vi "readLOG.vi"() -> ()   [LabVIEW 2011]
uses:
  <vilib>/Utility/file.llb/Write To Spreadsheet File (DBL).vi
panel:
  in  "save":bool
  out "output cluster":cluster{i32[], dbl[]}[](graph)=[{[0, 1, 2, 3, 4, 5, 6, 7, 8, 9, 10, 11, 12, 13, 14, 15, 16, 17, 18, 19, 20, 21, 22, 23, 24, 25, 26, 27, 28, 29, 30, 31, 32, 33, 34, 35, 36, 37, 38, 39, 40, 41, 42, 43, 44, 45, 46, 47, 48, 49, 50, 51, 52, 53, 54, 55, 56, 57, 58, 59, 60, 61, 62, 63, 64, 65, 66, 67, 68, 69, 70, 71, 72, 73, 74, 75, 76, 77, 78, 79, 80, 81, 82, 83, 84, 85, 86, 87, 88, 89, 90, 91, 92, 93, 94, 95, 96, 97, 98, 99, 100, 101, 102, 103, 104, 105, 106, 107, 108, 109, 110, 111, 112, 113, 114, 115, 116, 117, 118, 119, 120, 121, 122, 123, 124, 125, 126, 127, 128, 129, 130, 131, 132, 133, 134, 135, 136, 137, 138, 139, 140, 141, 142, 143, 144, 145, 146, 147, 148, 149, 150, 151, 152, 153, 154, 155, 156, 157, 158, 159, 160, 161, 162, 163, 164, 165, 166, 167, 168, 169, 170, 171, 172, 173, 174, 175, 176, 177, 178, 179, 180, 181, 182, 183, 184, 185, 186, 187, 188, 189, 190, 191, 192, 193, 194, 195, 196, 197, 198, 199, 200, 201, 202, 203, 204, 205, 206, 207, 208, 209, 210, 211, 212, 213, 214, 215, 216, 217, 218, 219, 220, 221, 222, 223, 224, 225, 226, 227, 228, 229, 230, 231, 232, 233, 234, 235, 236, 237, 238, 239, 240, 241, 242, 243, 244, 245, 246, 247, 248, 249, 250, 251, 252, 253, 254, 255, 256, 257, 258, 259, 260, 261, 262, 263, 264, 265, 266, 267, 268, 269, 270, 271, 272, 273, 274, 275, 276, 277, 278, 279, 280, 281, 282, 283, 284, 285, 286, 287, 288, 289, 290, 291, 292, 293, 294, 295, 296, 297, 298, 299, 300, 301, 302, 303, 304, 305, 306, 307, 308, 309, 310, 311, 312, 313, 314, 315, 316, 317, 318, 319, 320, 321, 322, 323, 324, 325, 326, 327, 328, 329, 330, 331, 332, 333, 334, 335, 336, 337, 338, 339, 340, 341, 342, 343, 344, 345, 346, 347, 348, 349, 350, 351, 352, 353, 354, 355, 356, 357, 358, 359, 360, 361, 362, 363, 364, 365, 366, 367, 368, 369, 370, 371, 372, 373, 374, 375, 376, 377, 378, 379, 380, 381, 382, 383, 384, 385, 386, 387, 388, 389, 390, 391, 392, 393, 394, 395, 396, 397, 398, 399, 400, 401, 402, 403, 404, 405, 406, 407, 408, 409, 410, 411, 412, 413, 414, 415, 416, 417, 418, 419, 420, 421, 422, 423, 424, 425, 426, 427, 428, 429, 430, 431, 432, 433, 434, 435, 436, 437, 438, 439, 440, 441, 442, 443, 444, 445, 446, 447, 448, 449, 450, 451, 452, 453, 454, 455, 456, 457, 458, 459, 460, 461, 462, 463, 464, 465, 466, 467, 468, 469, 470, 471, 472, 473, 474, 475, 476, 477, 478, 479, 480, 481, 482, 483, 484, 485, 486, 487, 488, 489, 490, 491, 492, 493], [nan, nan, nan, nan, nan, nan, nan, nan, nan, nan, nan, nan, nan, nan, nan, nan, nan, nan, nan, nan, nan, nan, nan, nan, nan, nan, nan, nan, nan, nan, nan, nan, nan, nan, nan, nan, nan, nan, nan, nan, nan, nan, nan, nan, nan, nan, nan, nan, nan, nan, nan, nan, nan, nan, nan, nan, nan, nan, nan, nan, nan, nan, nan, nan, nan, nan, nan, nan, nan, nan, nan, nan, nan, nan, nan, nan, nan, nan, nan, nan, nan, nan, nan, nan, nan, nan, nan, nan, nan, nan, nan, nan, nan, nan, nan, nan, nan, nan, nan, nan, nan, nan, nan, nan, nan, nan, nan, nan, nan, nan, nan, nan, nan, nan, nan, nan, nan, nan, nan, nan, nan, nan, nan, nan, nan, nan, nan, nan, nan, nan, nan, nan, nan, nan, nan, nan, nan, nan, nan, nan, nan, nan, nan, nan, nan, nan, nan, nan, nan, nan, nan, nan, nan, nan, nan, nan, nan, nan, nan, nan, nan, nan, nan, nan, nan, nan, nan, nan, nan, nan, nan, nan, nan, nan, nan, nan, nan, nan, nan, nan, nan, nan, nan, nan, nan, nan, nan, nan, nan, nan, nan, nan, nan, nan, nan, nan, nan, nan, nan, nan, nan, nan, nan, nan, nan, nan, nan, nan, nan, nan, nan, nan, nan, nan, nan, nan, nan, nan, nan, nan, nan, nan, nan, nan, nan, nan, nan, nan, nan, nan, nan, nan, nan, nan, nan, nan, nan, nan, nan, nan, nan, nan, nan, nan, nan, nan, nan, nan, nan, nan, nan, nan, nan, nan, nan, nan, nan, nan, nan, nan, nan, nan, nan, nan, nan, nan, nan, nan, nan, nan, nan, nan, nan, nan, nan, nan, nan, nan, nan, nan, nan, nan, nan, nan, nan, nan, nan, nan, nan, nan, nan, nan, nan, nan, nan, nan, nan, nan, nan, nan, nan, nan, nan, nan, nan, nan, nan, nan, nan, nan, nan, nan, nan, nan, nan, nan, nan, nan, nan, nan, nan, nan, nan, nan, nan, nan, nan, nan, nan, nan, nan, nan, nan, nan, nan, nan, nan, nan, nan, nan, nan, nan, nan, nan, nan, nan, nan, nan, nan, nan, nan, nan, nan, nan, nan, nan, nan, nan, nan, nan, nan, nan, nan, nan, nan, nan, nan, nan, nan, nan, nan, nan, nan, nan, nan, nan, nan, nan, nan, nan, nan, nan, nan, nan, nan, nan, nan, nan, nan, nan, nan, nan, nan, nan, nan, nan, nan, nan, nan, nan, nan, nan, nan, nan, nan, nan, nan, nan, nan, nan, nan, nan, nan, nan, nan, nan, nan, nan, nan, nan, nan, nan, nan, nan, nan, nan, nan, nan, nan, nan, nan, nan, nan, nan, nan, nan, nan, nan, nan, nan, nan, nan, nan, nan, nan, nan, nan, nan, nan, nan, nan, nan, nan, nan, nan, nan, nan, nan, nan, nan, nan, nan, nan, nan, nan, nan, nan, nan, nan, nan, nan, nan, nan, nan, nan, nan, nan, nan, nan, nan, nan, nan, nan, nan, nan, nan, nan, nan, nan, nan, nan, nan, nan, nan]}, {[0, 1, 2, 3, 4, 5, 6, 7, 8, 9, 10, 11, 12, 13, 14, 15, 16, 17, 18, 19, 20, 21, 22, 23, 24, 25, 26, 27, 28, 29, 30, 31, 32, 33, 34, 35, 36, 37, 38, 39, 40, 41, 42, 43, 44, 45, 46, 47, 48, 49, 50, 51, 52, 53, 54, 55, 56, 57, 58, 59, 60, 61, 62, 63, 64, 65, 66, 67, 68, 69, 70, 71, 72, 73, 74, 75, 76, 77, 78, 79, 80, 81, 82, 83, 84, 85, 86, 87, 88, 89, 90, 91, 92, 93, 94, 95, 96, 97, 98, 99, 100, 101, 102, 103, 104, 105, 106, 107, 108, 109, 110, 111, 112, 113, 114, 115, 116, 117, 118, 119, 120, 121, 122, 123, 124, 125, 126, 127, 128, 129, 130, 131, 132, 133, 134, 135, 136, 137, 138, 139, 140, 141, 142, 143, 144, 145, 146, 147, 148, 149, 150, 151, 152, 153, 154, 155, 156, 157, 158, 159, 160, 161, 162, 163, 164, 165, 166, 167, 168, 169, 170, 171, 172, 173, 174, 175, 176, 177, 178, 179, 180, 181, 182, 183, 184, 185, 186, 187, 188, 189, 190, 191, 192, 193, 194, 195, 196, 197, 198, 199, 200, 201, 202, 203, 204, 205, 206, 207, 208, 209, 210, 211, 212, 213, 214, 215, 216, 217, 218, 219, 220, 221, 222, 223, 224, 225, 226, 227, 228, 229, 230, 231, 232, 233, 234, 235, 236, 237, 238, 239, 240, 241, 242, 243, 244, 245, 246, 247, 248, 249, 250, 251, 252, 253, 254, 255, 256, 257, 258, 259, 260, 261, 262, 263, 264, 265, 266, 267, 268, 269, 270, 271, 272, 273, 274, 275, 276, 277, 278, 279, 280, 281, 282, 283, 284, 285, 286, 287, 288, 289, 290, 291, 292, 293, 294, 295, 296, 297, 298, 299, 300, 301, 302, 303, 304, 305, 306, 307, 308, 309, 310, 311, 312, 313, 314, 315, 316, 317, 318, 319, 320, 321, 322, 323, 324, 325, 326, 327, 328, 329, 330, 331, 332, 333, 334, 335, 336, 337, 338, 339, 340, 341, 342, 343, 344, 345, 346, 347, 348, 349, 350, 351, 352, 353, 354, 355, 356, 357, 358, 359, 360, 361, 362, 363, 364, 365, 366, 367, 368, 369, 370, 371, 372, 373, 374, 375, 376, 377, 378, 379, 380, 381, 382, 383, 384, 385, 386, 387, 388, 389, 390, 391, 392, 393, 394, 395, 396, 397, 398, 399, 400, 401, 402, 403, 404, 405, 406, 407, 408, 409, 410, 411, 412, 413, 414, 415, 416, 417, 418, 419, 420, 421, 422, 423, 424, 425, 426, 427, 428, 429, 430, 431, 432, 433, 434, 435, 436, 437, 438, 439, 440, 441, 442, 443, 444, 445, 446, 447, 448, 449, 450, 451, 452, 453, 454, 455, 456, 457, 458, 459, 460, 461, 462, 463, 464, 465, 466, 467, 468, 469, 470, 471, 472, 473, 474, 475, 476, 477, 478, 479, 480, 481, 482, 483, 484, 485, 486, 487, 488, 489, 490, 491, 492, 493], [nan, nan, nan, 14.066518781879608, 13.6877666266289, 13.503670363706988, nan, 13.753226441574611, 13.424672107298193, 13.060270267975284, nan, nan, 13.013151223607906, 13.827191090757537, 14.096268945337101, 13.881347076649377, 13.835007846379085, 14.029751029979366, 14.558635788659672, 14.568579824747644, 14.745564055289833, 14.681206964257171, 14.807516860214946, 15.097728499268555, 15.127994983609142, 15.38337156947, 15.394784866334476, 15.647507607601483, 15.747405526777243, 15.688804480557906, 15.735395542988613, 15.81766743931928, 16.003685961275778, 15.838374148868525, nan, 15.661872710887451, 16.032722041258808, 15.895152587914822, 16.507018771049047, 16.10779669753117, 14.535536931781962, 15.917051760046434, 16.351400826697386, 16.331351226114748, 16.582203344567347, 16.93608575913413, 16.623143378740565, 16.464115878746497, 16.32701081848836, 16.843980765385027, 16.637401617612227, 16.412354436417786, 15.085569734480714, 16.25351262356935, 16.993151552608083, 16.735036841620172, 16.951045490536217, 16.328951032958344, 16.446609143863498, 16.355403131910407, 16.677847066531285, 16.71186124920689, 16.683893236888025, 16.670427878227883, 16.607700114039403, 16.77322991473443, 17.234557000901987, 16.674907349503542, 16.739306265224513, 11.984522358485037, 16.995092296674557, 17.2025886141937, 17.019183414148415, 16.990302706290095, 17.40012777421066, 16.93419344163351, 17.52475415049969, 17.738712218766977, 17.782635888950722, 17.15761490297507, 17.313055402015948, 17.083861665444715, 17.95258358856597, 17.48207497621911, 17.751917173582342, 17.732699069261344, 16.220493880144318, 18.091232313654928, 18.28496658271297, 17.74773835952726, 18.038872316356787, 16.815928573646943, 17.83465375820458, 18.000002216927896, 17.97775576956883, 17.982941936926977, 18.02713108065234, 18.181385226176985, 15.261310888524008, 16.81114156771639, 18.001059406042373, 17.88088451812689, 18.084194751920677, 18.299314104207156, 18.108866561806508, 18.36302034657365, 18.45917382818027, 18.724189534745847, 18.010434003954288, 18.310388405488084, 18.10850920741916, 18.6681765452264, 18.338547313820413, 18.148235101326577, 15.755307273780431, 16.503291290419952, 16.427608587956684, nan, nan, nan, nan, nan, nan, nan, nan, nan, nan, nan, nan, nan, 16.832484778315802, 17.301460607229956, 17.861757877778814, 17.315890374469063, 18.387846340229657, 18.44911782087206, 18.299613630144677, 18.063320964964646, nan, 18.210816856054066, 18.07321283068086, 15.942788561682391, 18.530383799112656, 18.172768588804843, 17.17467713959809, 18.20392031492156, 18.218647186515568, 18.318049215139695, 18.461975329057054, 18.49546892899582, 18.563761083530494, 18.39510878522958, 18.373880645364807, 18.82213149911786, 18.54667405049622, 18.807521443681253, 19.04184200162115, 13.948488087858664, 18.947112380012527, 18.894829681565966, 19.01661398003887, 18.899081320819278, 15.40293481834965, 19.134471446204657, 16.748170723655562, 19.321879182996327, 19.249424354413577, 19.54227394418865, 19.4095924077086, 19.570741551015203, 19.39690241471874, 19.47355015471669, 19.635747032950235, 19.583844173957687, 19.301091873203177, 19.64877382242514, 19.727852179608817, 19.92196497701559, 19.94014110498813, 16.06848583723081, 20.037571800516957, 19.822544441395394, 19.955990306032163, 19.730445683905714, 19.688940234178062, 19.840538766819463, 19.94058600910762, 19.848167235801156, 20.11460928834606, 20.287658747560272, 20.114678068272156, 20.15604184819108, 20.179767884061334, 20.1887297914825, 20.22797984119802, 18.829274035823232, 20.193669192157813, 20.281480661493106, 18.92553790894135, 20.012316075332933, 20.326906879062676, 20.41794080217153, 20.270067276330337, 20.38020878217344, 20.44943979384732, 20.417626169446066, 20.694222242962724, 20.58853148061519, 20.532936145612666, 20.516188577090816, 20.912152265605755, 20.72704101160798, 20.548038887925713, 19.47660759434541, 18.268746257227917, 19.407708129163893, 19.230888431381345, 20.456508111369317, 20.89990402732053, 20.73211377913094, 21.083096448822744, 20.859749688853867, 20.804908290215394, 20.90965144046322, 20.992284607532156, 21.117201166386963, 21.076462222309033, 21.161555779557602, 20.821636956847783, 20.99488454769221, 21.26157849707056, 21.380503240714688, 21.136905930661214, 21.059126899764237, 21.306537133427128, 21.33329493568783, 21.38027102831404, 21.35114902954888, 21.244195587005493, 21.473746016599193, 21.447810346679717, 21.379628744501815, 21.10973930598732, 21.58049338336491, 18.943231684453963, 21.469805722950014, 21.70789372848526, 21.30058796700473, 21.99258945848294, 21.72341755880302, 21.447983719322792, 21.767859751820424, 21.73517503218727, 21.702637543497644, 21.608946394004533, 21.718036298291395, 21.840109465538717, 21.839714270861805, 21.981872745804708, 21.993840877182038, 21.957183060839043, 21.802370723057606, 21.88013599540841, 19.319235956480043, 21.830957740379972, 21.87484922046849, 21.80714143209468, 19.48552134830811, 22.034493248465196, 21.97763594105436, 21.677775655800474, 21.93313481341204, 21.98388516943089, 22.000399181565058, 18.325648850669268, 22.04614514540924, 22.106541329599054, 22.016559561043437, 22.053810663685226, 22.006609576691403, 21.72275753294673, 18.776248930419797, 22.31017594705952, 22.249144514321756, 18.772478024340558, 22.19852119564098, 22.498126596662246, 22.365816132794862, 22.326614032657858, 22.482123002840353, 21.237214090313273, 22.602090457727627, 22.52128600481194, 22.471070924311334, 22.51707587539738, 22.416871656350736, 22.505478131942937, 22.564612779302024, 22.61655930910456, 22.975177120821854, 22.640932813517338, 22.80095861183122, 22.66092894385099, 22.796680037271926, 19.30723952923904, 22.55504104016302, 22.54053494708512, 22.73666472546904, 22.79059570567847, 22.784559444658157, 22.727199161315184, 22.651254431484517, 22.807342100175106, 22.99505130984835, 23.109871449084153, 23.167885623747566, 23.256039159683382, 23.24296460266214, 23.172805402968493, 17.956881538133757, 21.99279344885008, 23.1284683630887, 23.405176338326896, 23.21177057348541, nan, 23.128359288722095, 23.44326842266196, 23.535134091836767, 23.312073479128685, 23.3895110104271, 23.662200416275482, 23.475803780147885, 23.059776716849115, 23.28254766790917, 23.444643098647134, 23.265680227575672, 23.44991076846179, 23.43486851191858, 23.353569411265426, 23.56149436758062, 23.419723476046215, 23.5804266106893, 23.581193808425496, 23.570602863972, 23.728141191605346, 18.418851805196823, 23.807396946693302, 23.6508460979785, 23.561716368113707, 23.593473553452668, 23.805798851148666, 23.596698224294073, 22.444582918994683, 23.8231787149341, 23.81920986463558, 23.71260065415538, 22.55683076462867, 23.80720622756246, 23.690627562811756, 23.638593381945043, 23.558214624504103, 23.679329596103912, 23.753965676444636, 23.717202098171356, 23.990662638950766, 23.763852242795792, 18.8964874693271, 22.549364936054758, 23.98456660237275, 23.986546118434035, 23.871256765607768, 24.071946783301314, 23.849630482108523, 22.837140826571158, 24.068846378416083, 23.980214611824977, 23.812700241238986, 23.910225553316536, 24.08346509262003, 24.006956830548347, 22.689022043814248, 24.015496187614417, 24.076411938152887, 21.56581794208114, 24.081698153358502, 24.07028578074096, 24.061245455642847, 24.315035912587064, 24.102320335125796, 24.027469531329416, 24.119355358647795, 24.523178672803056, 24.15586034198725, 24.256857294221163, 19.13640861275303, 24.086114772493715, 24.380147369661017, 21.817243477789475, 24.593974631887818, 23.930434860600826, 24.292534436745086, 24.296349846132102, 23.13597927021044, 24.591632925750787, 24.604790238716305, 24.637466954020965, 24.54440412249585, 24.23311749941149, 24.5309750390378, nan, 24.61553540409284, 24.81890691828835, 23.32350605062311, 24.446423761438496, 23.072715522621138, 24.70491730520837, 24.884465406247045, 24.624714184233426, 24.689671960039277, 24.650016905452958, 24.662732314264986, 24.679261827501023, 24.82550015212746, 23.49646809859314, 24.93428853502064, 24.92142239838165, 25.03947237554837, 24.783319985831213, 24.983066219615807, 24.953836022233418, 24.62492147313651, 24.830078945657647, 24.924997982460923, 24.629355324681228, 24.661710943505454, 24.610488392856723, 24.834232003746592, 25.011810055014166, 25.060728478488386, 24.83233638359627, 25.21472203545045, 25.09920816734268, 25.07141796561291, 24.92445278850198, 19.666016715228807, 23.674784033613037, 24.680256548898228, 25.297027373102537, 25.090705007730662, 25.055673179691325, 22.403396363598745, 25.112785818503994, 25.385898530466875, 24.845410704591586, 25.274103228689683, 25.47277074264889, 20.052714772838044, 25.289432980773768, 25.103268061909944, 25.421086306184066, 25.365803267457068, 25.268317180999134, 25.322264043173163, 25.349575147905284, 25.44863008584025, 23.984885099462304, 25.483122918636013, 25.15604508413594, 25.110654221636082, 25.27800312625027, 24.12203582790778, 25.635494716883386, 25.534693292755264, 23.057821878265486, 25.522154124926942, 25.51254296564332, 25.596429219776496, 25.684348019114168, 25.333276618155992, 25.731105837604446, 25.580961168395334, 18.153913292885136, 24.62196905754581, 25.6704439385054, 25.910264096158812, 25.45606884180677, 25.433030895008073, 25.94672384763146, 25.82463205289241, 25.813436309984922, 25.560540253058775, 25.524152796836916, 25.82532067897364, 25.638865199291786]}, {[0, 1, 2, 3, 4, 5, 6, 7, 8, 9, 10, 11, 12, 13, 14, 15, 16, 17, 18, 19, 20, 21, 22, 23, 24, 25, 26, 27, 28, 29, 30, 31, 32, 33, 34, 35, 36, 37, 38, 39, 40, 41, 42, 43, 44, 45, 46, 47, 48, 49, 50, 51, 52, 53, 54, 55, 56, 57, 58, 59, 60, 61, 62, 63, 64, 65, 66, 67, 68, 69, 70, 71, 72, 73, 74, 75, 76, 77, 78, 79, 80, 81, 82, 83, 84, 85, 86, 87, 88, 89, 90, 91, 92, 93, 94, 95, 96, 97, 98, 99, 100, 101, 102, 103, 104, 105, 106, 107, 108, 109, 110, 111, 112, 113, 114, 115, 116, 117, 118, 119, 120, 121, 122, 123, 124, 125, 126, 127, 128, 129, 130, 131, 132, 133, 134, 135, 136, 137, 138, 139, 140, 141, 142, 143, 144, 145, 146, 147, 148, 149, 150, 151, 152, 153, 154, 155, 156, 157, 158, 159, 160, 161, 162, 163, 164, 165, 166, 167, 168, 169, 170, 171, 172, 173, 174, 175, 176, 177, 178, 179, 180, 181, 182, 183, 184, 185, 186, 187, 188, 189, 190, 191, 192, 193, 194, 195, 196, 197, 198, 199, 200, 201, 202, 203, 204, 205, 206, 207, 208, 209, 210, 211, 212, 213, 214, 215, 216, 217, 218, 219, 220, 221, 222, 223, 224, 225, 226, 227, 228, 229, 230, 231, 232, 233, 234, 235, 236, 237, 238, 239, 240, 241, 242, 243, 244, 245, 246, 247, 248, 249, 250, 251, 252, 253, 254, 255, 256, 257, 258, 259, 260, 261, 262, 263, 264, 265, 266, 267, 268, 269, 270, 271, 272, 273, 274, 275, 276, 277, 278, 279, 280, 281, 282, 283, 284, 285, 286, 287, 288, 289, 290, 291, 292, 293, 294, 295, 296, 297, 298, 299, 300, 301, 302, 303, 304, 305, 306, 307, 308, 309, 310, 311, 312, 313, 314, 315, 316, 317, 318, 319, 320, 321, 322, 323, 324, 325, 326, 327, 328, 329, 330, 331, 332, 333, 334, 335, 336, 337, 338, 339, 340, 341, 342, 343, 344, 345, 346, 347, 348, 349, 350, 351, 352, 353, 354, 355, 356, 357, 358, 359, 360, 361, 362, 363, 364, 365, 366, 367, 368, 369, 370, 371, 372, 373, 374, 375, 376, 377, 378, 379, 380, 381, 382, 383, 384, 385, 386, 387, 388, 389, 390, 391, 392, 393, 394, 395, 396, 397, 398, 399, 400, 401, 402, 403, 404, 405, 406, 407, 408, 409, 410, 411, 412, 413, 414, 415, 416, 417, 418, 419, 420, 421, 422, 423, 424, 425, 426, 427, 428, 429, 430, 431, 432, 433, 434, 435, 436, 437, 438, 439, 440, 441, 442, 443, 444, 445, 446, 447, 448, 449, 450, 451, 452, 453, 454, 455, 456, 457, 458, 459, 460, 461, 462, 463, 464, 465, 466, 467, 468, 469, 470, 471, 472, 473, 474, 475, 476, 477, 478, 479, 480, 481, 482, 483, 484, 485, 486, 487, 488, 489, 490, 491, 492, 493], [nan, nan, nan, 5.838373005935011, 5.122962592515421, 4.495991600341085, nan, 6.284850197128378, 6.772034070844995, 8.86161842766137, nan, nan, 10.119567234038982, 6.24472172053288, 7.333369065432976, 10.842566631747047, 10.71901156161698, 9.139639127103749, 8.136834081536165, 8.611732281336344, 6.900357273426437, 5.825207630283842, 12.417107534156344, 6.3508136501162085, 9.427983233683904, 7.84821697929641, 9.805387578457612, 8.94038871321834, 11.92743483200735, 10.4262763810612, 9.169585527257084, 10.200337314738931, 11.223305444495395, 10.142130031813565, nan, 6.087129327291905, 9.69613494127924, 8.920700640346183, 12.313869321080574, 8.048223109615776, 5.869274016395934, 7.258172149814584, 6.144714568212578, 6.167343587115909, 7.228882446185537, 10.303585183441783, 8.384095390592563, 7.0122251051909075, 5.570601349678213, 9.030386710849882, 6.9734479791717945, 5.628446949880868, 5.702900496986786, 7.523414765339112, 5.414394477101268, 5.66046410096169, 5.129551113776415, 4.667133729356067, 6.326430976798406, 4.992043274279808, 5.927780831679172, 5.277571283119926, 5.6776772648937595, 5.380436131576687, 5.985308939617596, 4.426722949332543, 8.487393998998698, 4.894050305144333, 4.786741239679316, 6.33374532263764, 5.053858786821195, 5.29592669672428, 4.567352635691293, 5.153821563506028, 5.848178761645272, 4.754057801738497, 8.132698272434027, 6.456074483018654, 5.835539041387904, 4.117962741222755, 5.421742906376608, 4.077895993348989, 7.366806393861509, 6.374268874915856, 5.511027175308186, 6.377641016515611, 4.0120261023465105, 7.11601258777614, 8.455913051814889, 5.630230454023035, 6.240651201189905, 7.360327549907083, 4.095103095691115, 5.629870587679363, 5.41037635068227, 5.478495412809252, 5.391712393021919, 5.291224065810866, 4.941623696735348, 5.101579449837175, 4.699076657353999, 4.0275985269285, 4.869064921934353, 4.344990175234898, 4.062861272941063, 6.208364384085257, 5.787023238139568, 5.320211812781167, 3.752695395322746, 5.123256594596057, 4.478564715942355, 4.545455970980356, 4.42642406105557, 6.273310263435405, 4.062187187512961, 4.039394078824671, 5.137740161042757, 4.550444389342431, 5.201665366816314, 5.324430156220558, 4.994665423442655, 5.095640161687982, 4.5627074926381965, 4.992444393130484, 4.655358355386113, 3.1755203314531855, 2.680678202758031, 5.149211642121998, 4.772676978731226, 5.30809161178945, 3.8855565150530538, 2.0588444130228254, 3.6764625595305915, 2.929531871688198, 4.618848705134042, 4.640622483393713, 5.062929475088538, 5.0967879023218075, nan, 2.5480877774244277, 4.9806954984139225, 6.139215940084341, 4.933652505056159, 5.2192525568939345, 5.651965608860735, 4.462021637293276, 4.90738852457622, 5.2234311401724085, 4.5061080302521646, 4.9864354628487035, 5.172546314348892, 5.224734656061742, 5.279041764629142, 3.9407082282950228, 4.312976132425604, 5.191142359253661, 4.819403956011911, 4.971310632950292, 5.065820113080008, 5.631097100654131, 5.554126212247638, 5.099662880102869, 4.2951034283975105, 4.952621809954223, 5.135941423772067, 6.33029925635708, 5.2439017049412655, 5.267807885769059, 4.908985559321138, 4.680428811755689, 7.025725350173275, 5.377854731837658, 5.482157076237286, 5.733883331449249, 5.59656472178699, 4.97666287286728, 5.285608725421014, 8.118542449436745, 5.1289913421171605, 6.291890043818455, 4.987848174930832, 6.067430883766349, 5.59679965051788, 6.358313205852653, 5.732344746654803, 6.078315867420372, 6.257439015679154, 6.460738654642967, 7.4692176243733, 6.360715012493415, 6.195447029201148, 6.304687743200418, 4.858125278037562, 5.573466305008537, 6.355279777663554, 5.937668851479032, 7.115418978520438, 6.901683985799764, 6.498390921819009, 2.8056970509927623, 5.776727225705713, 4.877154979161503, 7.614503024663179, 6.5725564834500005, 6.9997664257659835, 7.363856180122184, 6.807954704047688, 6.467988948787763, 6.94286601725355, 6.754464303271163, 6.758434146805712, 6.393922049849095, 6.604244797106844, 7.0418976452521065, 7.169857290373443, 6.737737284289949, 4.140756370887686, 3.9221909690363077, 6.593770619997429, 6.8855523095336935, 7.499117068436192, 7.842313028945739, 7.5164783493946175, 7.797339867943151, 7.794903103621948, 7.3494156610997265, 7.201164679096905, 8.835886252056582, 9.270272944038197, 8.02114409404902, 7.317043750826599, 9.46362569728808, 7.647850083636058, 7.641421356725573, 8.678143614429189, 8.098861409126641, 8.211312934802379, 9.439975564734993, 7.889815992253432, 8.617290550361588, 8.921648020827035, 8.439333164258358, 6.606140105055147, 8.466598412839062, 8.39636887605917, 8.93351449020821, 7.8432078071359115, 5.8409437250793985, 8.524941464460937, 9.0945326721004, 8.522435306711259, 9.248171396795215, 9.196036237964279, 9.216838801941833, 8.569081296371962, 9.619347038846172, 10.677497642324852, 7.989271148128637, 8.258189152667683, 9.280954711393349, 9.190808358636218, 9.140827295923543, 9.130850235144067, 9.919454819340388, 9.471843595812288, 10.269642908893047, 9.694510920632467, 9.80501148024473, 9.361651188055475, 9.987097544496066, 6.825297282127792, 8.679616545630324, 9.619432193623538, 9.53942192987705, 9.170668461395962, 9.651344279937518, 9.454641713828494, 9.182247245284543, 9.667341123407198, 9.044768016601779, 5.007807912381509, 9.485305211565674, 9.810683905852784, 9.893023157703453, 9.427293919586816, 10.10503077720574, 10.256211644359041, 8.580460000201697, 9.335644622849088, 8.7587075374135, 9.270035331225415, 10.291678353814916, 10.264348564835643, 10.325497901662345, 10.07986676691985, 10.174339048017316, 11.025732557259857, 10.269462664848163, 7.850156871642014, 9.950903507641328, 10.992304308241216, 10.637087946189524, 10.865463896206165, 11.110381603269673, 10.321796090014914, 10.37792582642129, 11.397671541639056, 10.555248675961252, 10.499060363401384, 10.78327867922934, 10.497836854920138, 12.130529772736168, 10.913351302325736, 11.196379705849267, 11.086087086130703, 12.236093656989624, 10.890200394884914, 10.909049510928185, 11.56994998931583, 11.08676449101506, 11.308383099740013, 12.906205258621128, 11.422300898148876, 12.110139887947298, nan, 11.152329704668944, 11.281840525154792, 11.231996424652834, 12.215759393799317, 12.711731259545843, 11.618627690461437, 12.266100594166346, 10.70585326563372, 13.68243887841669, 11.860010265208416, 12.243250988406885, 12.347211871006607, 12.094146355336477, 11.323535343670414, 12.573563063585198, 12.22446516449071, 13.198342509771521, 13.34346677698494, 12.422345078756962, 13.331231387210096, 12.923114844427516, 12.28054246880447, 12.267719283646557, 12.631091802582034, 13.48780413989192, 12.037870786815972, 12.809537453537814, 12.3794812876626, 12.08315040813875, 12.177166186131728, 12.898433742365, 13.516993211907788, 12.527109955478807, 12.616895181824702, 12.722840046287274, 11.727814226434646, 11.425213856734558, 12.614595996659432, 16.111345754512513, 12.085848561733485, 13.663474987635084, 13.02591233375847, 12.79626656894743, 12.987456668638345, 12.60081629948587, 12.17447435518676, 12.913905199960652, 13.962035187071365, 13.699538782696038, 12.870127240945578, 13.010583248384762, 12.95703557057658, 12.86294828321337, 12.633219719355168, 13.316984224468627, 13.220971182770938, 13.09025324012299, 12.439590014514465, 11.955877858767394, 14.98695287863086, 12.162141525533684, 14.017980881062272, 12.111376446199074, 13.84290426884371, 13.533596503302306, 12.57054937820601, 12.465144568211088, 13.399528504285172, 12.732660098370843, 12.318810326626988, 12.67198278820382, 12.349270165341807, 13.534416623121842, 12.01150270059884, 13.838151740458557, 12.683154026358125, 13.347591373273417, 12.356935502410977, 12.31374461238488, 12.478775010862876, 12.997842969109968, 12.911354469227604, 14.243574875580862, 12.76897240974938, nan, 12.626898535493979, 12.394720022265517, 12.85352616355857, 13.166796774354168, 13.103343737752425, 13.103204324169951, 13.887718613743402, 13.194476451958678, 13.136160754762443, 12.121751664383169, 11.766080753165454, 12.533367788410487, 11.81251317477745, 12.12844139533587, 12.064360779600293, 12.81931333871779, 11.887057517100118, 12.201858732994197, 11.768313429933869, 12.534648373860819, 12.5981318444654, 11.707357661619312, 11.261032845422903, 13.662119453875391, 11.53368270044183, 12.220301920337022, 12.589947321118245, 11.417726238526825, 11.680761956899573, 12.627646519022562, 11.938575785404225, 12.235449602579934, 12.359900855294313, 13.006779528886682, 11.435209291301419, 12.264056380942407, 12.413466357464529, 11.144559733160236, 11.974540697212944, 12.47500752570079, 11.615848984345632, 14.642024451070142, 11.956265011371613, 12.984154222402026, 11.692847877350289, 12.132508718455881, 12.404938559579648, 12.39606080532883, 13.314117983568167, 12.54848851067078, 11.879753845363041, 12.509234473995434, 12.228053247995149, 13.616690008481726, 11.807865805091353, 12.309139015014182, 12.417092131102095, 11.926404908394261, 11.093656023162339, 12.482689678125666, 11.941869111918152, 11.925612507482526, 12.543853735254629, 11.867250443876173, 12.495516463649267, 13.361418214330286, 11.811194950868185, 12.514799932855567, 12.85696245258191, 11.526948542616537, 12.404799287606124, 12.490858627559419, 12.22245653013033, 12.267893030358039, 11.47370683628776, 13.205665356262841, 13.038580800760656, 12.457340648292416, 13.21341125707147, 12.30849104360999, 12.186694767560994, nan, 12.776164202755012, 13.230246294030337]}, {[0, 1, 2, 3, 4, 5, 6, 7, 8, 9, 10, 11, 12, 13, 14, 15, 16, 17, 18, 19, 20, 21, 22, 23, 24, 25, 26, 27, 28, 29, 30, 31, 32, 33, 34, 35, 36, 37, 38, 39, 40, 41, 42, 43, 44, 45, 46, 47, 48, 49, 50, 51, 52, 53, 54, 55, 56, 57, 58, 59, 60, 61, 62, 63, 64, 65, 66, 67, 68, 69, 70, 71, 72, 73, 74, 75, 76, 77, 78, 79, 80, 81, 82, 83, 84, 85, 86, 87, 88, 89, 90, 91, 92, 93, 94, 95, 96, 97, 98, 99, 100, 101, 102, 103, 104, 105, 106, 107, 108, 109, 110, 111, 112, 113, 114, 115, 116, 117, 118, 119, 120, 121, 122, 123, 124, 125, 126, 127, 128, 129, 130, 131, 132, 133, 134, 135, 136, 137, 138, 139, 140, 141, 142, 143, 144, 145, 146, 147, 148, 149, 150, 151, 152, 153, 154, 155, 156, 157, 158, 159, 160, 161, 162, 163, 164, 165, 166, 167, 168, 169, 170, 171, 172, 173, 174, 175, 176, 177, 178, 179, 180, 181, 182, 183, 184, 185, 186, 187, 188, 189, 190, 191, 192, 193, 194, 195, 196, 197, 198, 199, 200, 201, 202, 203, 204, 205, 206, 207, 208, 209, 210, 211, 212, 213, 214, 215, 216, 217, 218, 219, 220, 221, 222, 223, 224, 225, 226, 227, 228, 229, 230, 231, 232, 233, 234, 235, 236, 237, 238, 239, 240, 241, 242, 243, 244, 245, 246, 247, 248, 249, 250, 251, 252, 253, 254, 255, 256, 257, 258, 259, 260, 261, 262, 263, 264, 265, 266, 267, 268, 269, 270, 271, 272, 273, 274, 275, 276, 277, 278, 279, 280, 281, 282, 283, 284, 285, 286, 287, 288, 289, 290, 291, 292, 293, 294, 295, 296, 297, 298, 299, 300, 301, 302, 303, 304, 305, 306, 307, 308, 309, 310, 311, 312, 313, 314, 315, 316, 317, 318, 319, 320, 321, 322, 323, 324, 325, 326, 327, 328, 329, 330, 331, 332, 333, 334, 335, 336, 337, 338, 339, 340, 341, 342, 343, 344, 345, 346, 347, 348, 349, 350, 351, 352, 353, 354, 355, 356, 357, 358, 359, 360, 361, 362, 363, 364, 365, 366, 367, 368, 369, 370, 371, 372, 373, 374, 375, 376, 377, 378, 379, 380, 381, 382, 383, 384, 385, 386, 387, 388, 389, 390, 391, 392, 393, 394, 395, 396, 397, 398, 399, 400, 401, 402, 403, 404, 405, 406, 407, 408, 409, 410, 411, 412, 413, 414, 415, 416, 417, 418, 419, 420, 421, 422, 423, 424, 425, 426, 427, 428, 429, 430, 431, 432, 433, 434, 435, 436, 437, 438, 439, 440, 441, 442, 443, 444, 445, 446, 447, 448, 449, 450, 451, 452, 453, 454, 455, 456, 457, 458, 459, 460, 461, 462, 463, 464, 465, 466, 467, 468, 469, 470, 471, 472, 473, 474, 475, 476, 477, 478, 479, 480, 481, 482, 483, 484, 485, 486, 487, 488, 489, 490, 491, 492, 493], [nan, nan, nan, 24.25062821876577, 24.60133584212099, 24.325315160085665, nan, 25.21753593927707, 24.98777314753272, 25.35671035711158, nan, nan, 24.943638682249627, 25.342400016238457, 25.667555923599934, 25.413803698877985, 24.406811564950658, 24.67401192303828, 24.578851735407795, 24.678778061158198, 24.54719963880342, 24.46425825792153, 24.00829853676123, 24.5356710270558, 24.33173575978344, 24.640676534066813, 25.807277201152658, 25.496600317641594, 25.343325250347505, 24.927055281982632, 24.903586210834533, 25.963624932340053, 24.630070451184793, 24.689687517199218, nan, 26.632165975972157, 24.233498043703435, 24.691390331420337, 24.52135853923903, 25.184864766205294, 25.543664171336104, 24.999372428087213, 25.73927585174488, 25.916573153409445, 26.289984907221537, 25.414125665026404, 25.81550361777755, 25.72780887585259, 26.125390748133952, 25.78794804246661, 26.238241303462416, 26.582993889857164, 26.00122693876989, 24.90222411805871, 27.71568142375861, 27.655579844211502, 27.8830997759124, 27.204940978962497, 28.41078032727728, 27.013216608060873, 26.44500362546023, 26.67158726948196, 26.1288912414156, 26.596630580107217, 26.874876173170946, 27.584895720674297, 25.654663645304538, 26.523456041692214, 26.908834863502875, 26.675653218245486, 27.016018560213467, 27.153105355738944, 26.903462932391278, 26.04045487879671, 27.007705943216592, 26.998711376803044, 29.624295968676165, 26.042796140385747, 26.686810888877233, 27.416828943112932, 26.605300845173304, 27.146599836262112, 25.836812087495957, 27.929376646171477, 26.599457391652265, 26.251380820127793, 27.602491856725692, 26.604960937578824, 25.01842442669954, 26.44910076847765, 26.532547216648368, 25.22469072577968, 27.287599363796517, 26.889652783906968, 26.398699292158653, 27.01984582408147, 27.119652217303667, 26.953693620983586, 26.501167495992547, 26.541616247185175, 26.991874135613216, 26.12561788711514, 26.6354901081491, 27.21921071788711, 26.873737205274665, 26.635531638106045, 26.367033567511612, 26.27257692027962, 26.53583280978478, 26.5183797483985, 26.687011615803613, 27.10419027686646, 26.542539250988455, 27.49636973002572, 27.24285151262478, 26.8095365642356, 26.40885282212838, 26.348598960042466, 25.848767253724304, 26.247377004202008, 26.338299679258398, 26.039801561650677, 25.795633040589223, 26.324353279287777, 25.93143602271789, 26.277773426379326, 25.996978788946194, 25.97823748579316, 26.194693493799946, 25.74474614557107, 25.938236261414602, 26.22944198677112, 26.39423025325317, 25.541019714610172, 27.136897245270347, 26.42850053225243, 26.290222325220668, 25.5973844001727, nan, 25.643479396235477, 25.87440604971067, 25.380268238155168, 25.911454471001605, 25.69772485360113, 24.88667913163664, 25.156992122071188, 25.51230044009941, 25.634538233656258, 25.443590785583467, 25.040500644974145, 25.07158710840463, 24.85769811040859, 24.948057244801703, 25.678441885577854, 24.945428898638852, 25.278485261977835, 25.392813363952087, 25.208746342958875, 24.917412127313185, 26.373037415487943, 25.2439595173542, 25.017828400373105, 25.55095960433937, 25.632295002091155, 25.075420872957523, 25.153899677448862, 24.81406226839158, 24.62915827205353, 24.355919963132976, 24.861726160507658, 25.442700024093654, 24.607451977865196, 24.75240236829154, 24.72269150057957, 25.224286876391943, 25.65015229838241, 24.938624846230937, 27.78692778761672, 24.7899252010738, 25.494787739313153, 25.318032024278693, 24.52037733885652, 25.236413273119865, 25.254282578816913, 24.719600324325995, 24.4121420602184, 24.349414018447476, 24.49610633781782, 25.889178771467186, 24.60499995114361, 24.41394914442401, 24.902386183573697, 25.14381027700881, 24.641291170484408, 24.945094255917866, 26.094064714459194, 24.698615161176576, 24.695775604815026, 24.396231854567304, 24.686377081960757, 24.391407630466176, 24.475132931842893, 24.25692084028242, 24.571968791414918, 24.047895555311754, 23.945833110102797, 24.362024354288167, 24.050548346997687, 24.01678366088339, 23.164409206094035, 24.077973076424144, 23.940554403207273, 23.833389035649418, 23.971491276548136, 23.67246845411495, 23.44328243429061, 23.828259427161186, 23.58282988667048, 23.756695826028476, 22.98457997171988, 22.952134584054136, 22.743797268199785, 22.98027255082178, 23.44650526198899, 23.3966561805521, 22.987558572906437, 22.367613973963444, 24.564215225223904, 24.06664100467242, 22.802017343057514, 22.894254535364553, 24.79758792286634, 22.980893257270736, 23.860569816363295, 23.082367281147185, 22.75421508712708, 22.822212740568546, 24.051415884785115, 22.98446232262137, 24.711057737449266, 24.354691681411566, 23.266942134649298, 23.595314280439197, 23.629302056849497, 23.45788474220211, 22.725827905156564, 22.650699238640073, 24.33088973536468, 23.098213077448634, 22.708691717872853, 21.95035019242465, 22.05487862843148, 22.602212421397837, 22.726817289374083, 22.966010160274948, 24.13038549845055, 23.709333378104134, 23.173165259200744, 23.50031075349665, 25.355866812728607, 26.545058208753176, 24.025733599022203, 22.92173450802659, 21.662862210307026, 21.436060178281082, 21.160163934736545, 21.59083789708461, 21.86800033520001, 21.863543563080327, 21.538044630591514, 21.44946947254823, 21.525276756362302, 21.210709762176975, 22.512023096886196, 21.43656524355498, 21.185059888939293, 21.072924405898732, 20.721578606163803, 21.54673074178146, 21.600728320387077, 21.56200864699599, 21.770019387769196, 21.666868252530833, 21.66210519731345, 22.178427671662348, 21.558268681587435, 22.97516754137922, 21.834627020532082, 21.708588816624854, 21.747741980201965, 21.382643222988975, 21.72146705746576, 21.347936342570392, 21.076520127992296, 21.010327141878975, 20.64734197243257, 21.219681562661492, 21.247583173064868, 20.988831758927745, 21.89691185059644, 21.658561880557613, 21.76597653910119, 21.109143953666546, 20.927480018002996, 21.474557146945813, 21.331845449913715, 21.29633741406809, 21.808364535331123, 21.996967775501673, 21.41101176798486, 21.382663995942494, 22.526945431999934, 21.000004213218574, 22.5430886150657, 20.70978865123476, 22.462684238137, 21.05961973563103, 21.103736188575112, 21.06128637801646, 21.028746502914316, 21.423161755681804, 22.051798565576007, 21.151854336842746, 20.690577553839717, nan, 20.699281776745977, 20.775935534318535, 20.619300126933297, 20.457198658449556, 22.143220104913837, 21.49162475047183, 21.13024223163376, 20.546159334257823, 21.9735461711453, 20.62332629993648, 20.029636872159358, 20.391891906588683, 20.609054877427468, 20.246178980434138, 20.498503905262453, 20.637060336416937, 22.246288732269534, 22.525854504386018, 20.820735592446795, 22.1474662557128, 20.579976301527267, 20.73542197499205, 20.496149698954014, 20.462056231955557, 21.764130666208075, 20.552006921083148, 20.016935510755502, 20.30615266286071, 20.35272905404048, 20.335850689057622, 20.24260765797385, 21.23066933727773, 20.164203446186946, 20.280896422338856, 20.024171568762085, 19.847940985885714, 20.57095188937791, 20.339881456482487, 22.738127534405635, 20.287138418625375, 20.03666912131814, 20.262821447019064, 20.112221721100866, 20.094780533476865, 20.104892953799265, 19.54793716355033, 19.8386556376081, 20.838313858056154, 21.18750687452183, 20.098404428725928, 19.761786613918275, 19.339004131018612, 19.313041267699305, 19.711137785060203, 19.852932900967744, 19.69557404813071, 19.321177041110104, 19.509532793293772, 19.29424577206379, 21.95756947711476, 19.472124896869673, 20.68112612699133, 19.7053371747204, 20.586241604931274, 18.846178937895786, 19.004699758232846, 19.51545790020498, 18.92854607600907, 19.627433860370388, 19.32941992080754, 18.99656498215569, 19.54708991371109, 20.697965128324938, 19.731892833048107, 19.3774888586741, 19.775022622104473, 21.349262261269814, 19.483134012611004, 20.06838347710402, 19.824443891822227, 19.428025353737326, 18.959618263564153, 18.614065793420707, 18.95940189854082, nan, 19.284733815611105, 19.169651427913266, 19.17177945739536, 19.09635138629318, 18.41701339517624, 18.524959177117125, 20.07978951401384, 18.467642828786722, 18.59917344531067, 18.472008451862223, 18.710387359618153, 18.74738974946348, 18.5861197119753, 18.453020507883195, 18.007843377108088, 18.04194834988573, 18.89001079487042, 18.31990963790554, 18.79212953140751, 18.590554412895244, 18.14696147710049, 18.192624944075988, 18.324768643362916, 19.36046154647437, 18.12377205827869, 18.385315413142735, 18.30813784834976, 18.415963081817665, 18.102174965359495, 17.978235491579937, 18.11814111042304, 17.58392131105512, 18.011308146498436, 17.51450675899207, 17.708622815030992, 17.881455667484886, 17.122753861328704, 17.40923904107342, 16.79287299035383, 17.2340339551414, 17.221599829164404, 20.151729982771315, 17.82089099938429, 17.76551478177595, 17.697440422868965, 17.76493767780954, 17.86108375529426, 17.69159463411677, 17.285973829495333, 17.78612051716766, 17.92897011076468, 17.281782752549987, 17.692186824506905, 18.701569119118744, 17.55244187040438, 17.172869693455368, 16.992581186587017, 16.768848605648714, 16.89345331693636, 17.402949283211683, 17.45656748991769, 17.758450143227208, 17.6957007963548, 17.150540260366995, 17.180205128775924, 18.765683062629535, 17.306531394543526, 17.70349084378148, 17.271544816000187, 17.912534840887247, 17.92605866142344, 17.91836297287267, 17.734863352112427, 17.342562735690763, 17.57088111455181, 17.16168510057514, 16.94565189950106, 17.13625201751705, 18.541871668986516, 17.009535743738468, 17.344761961863185, nan, 17.19039842448649, 17.107927548941404]}, {[0, 1, 2, 3, 4, 5, 6, 7, 8, 9, 10, 11, 12, 13, 14, 15, 16, 17, 18, 19, 20, 21, 22, 23, 24, 25, 26, 27, 28, 29, 30, 31, 32, 33, 34, 35, 36, 37, 38, 39, 40, 41, 42, 43, 44, 45, 46, 47, 48, 49, 50, 51, 52, 53, 54, 55, 56, 57, 58, 59, 60, 61, 62, 63, 64, 65, 66, 67, 68, 69, 70, 71, 72, 73, 74, 75, 76, 77, 78, 79, 80, 81, 82, 83, 84, 85, 86, 87, 88, 89, 90, 91, 92, 93, 94, 95, 96, 97, 98, 99, 100, 101, 102, 103, 104, 105, 106, 107, 108, 109, 110, 111, 112, 113, 114, 115, 116, 117, 118, 119, 120, 121, 122, 123, 124, 125, 126, 127, 128, 129, 130, 131, 132, 133, 134, 135, 136, 137, 138, 139, 140, 141, 142, 143, 144, 145, 146, 147, 148, 149, 150, 151, 152, 153, 154, 155, 156, 157, 158, 159, 160, 161, 162, 163, 164, 165, 166, 167, 168, 169, 170, 171, 172, 173, 174, 175, 176, 177, 178, 179, 180, 181, 182, 183, 184, 185, 186, 187, 188, 189, 190, 191, 192, 193, 194, 195, 196, 197, 198, 199, 200, 201, 202, 203, 204, 205, 206, 207, 208, 209, 210, 211, 212, 213, 214, 215, 216, 217, 218, 219, 220, 221, 222, 223, 224, 225, 226, 227, 228, 229, 230, 231, 232, 233, 234, 235, 236, 237, 238, 239, 240, 241, 242, 243, 244, 245, 246, 247, 248, 249, 250, 251, 252, 253, 254, 255, 256, 257, 258, 259, 260, 261, 262, 263, 264, 265, 266, 267, 268, 269, 270, 271, 272, 273, 274, 275, 276, 277, 278, 279, 280, 281, 282, 283, 284, 285, 286, 287, 288, 289, 290, 291, 292, 293, 294, 295, 296, 297, 298, 299, 300, 301, 302, 303, 304, 305, 306, 307, 308, 309, 310, 311, 312, 313, 314, 315, 316, 317, 318, 319, 320, 321, 322, 323, 324, 325, 326, 327, 328, 329, 330, 331, 332, 333, 334, 335, 336, 337, 338, 339, 340, 341, 342, 343, 344, 345, 346, 347, 348, 349, 350, 351, 352, 353, 354, 355, 356, 357, 358, 359, 360, 361, 362, 363, 364, 365, 366, 367, 368, 369, 370, 371, 372, 373, 374, 375, 376, 377, 378, 379, 380, 381, 382, 383, 384, 385, 386, 387, 388, 389, 390, 391, 392, 393, 394, 395, 396, 397, 398, 399, 400, 401, 402, 403, 404, 405, 406, 407, 408, 409, 410, 411, 412, 413, 414, 415, 416, 417, 418, 419, 420, 421, 422, 423, 424, 425, 426, 427, 428, 429, 430, 431, 432, 433, 434, 435, 436, 437, 438, 439, 440, 441, 442, 443, 444, 445, 446, 447, 448, 449, 450, 451, 452, 453, 454, 455, 456, 457, 458, 459, 460, 461, 462, 463, 464, 465, 466, 467, 468, 469, 470, 471, 472, 473, 474, 475, 476, 477, 478, 479, 480, 481, 482, 483, 484, 485, 486, 487, 488, 489, 490, 491, 492, 493], [-240.39271255060729, -240.39271255060729, 8.607287449392715, 8.607287449392715, 8.607287449392715, 8.607287449392715, 8.607287449392715, 8.607287449392715, 8.607287449392715, 8.607287449392715, 7.6072874493927145, 7.6072874493927145, 7.6072874493927145, 7.6072874493927145, 8.607287449392715, 8.607287449392715, 7.6072874493927145, 7.6072874493927145, 8.607287449392715, 8.607287449392715, 8.607287449392715, 8.607287449392715, 7.6072874493927145, 8.607287449392715, 7.6072874493927145, 7.6072874493927145, 8.607287449392715, 7.6072874493927145, 7.6072874493927145, 7.6072874493927145, 7.6072874493927145, 7.6072874493927145, 7.6072874493927145, 7.6072874493927145, 7.6072874493927145, 8.607287449392715, 8.607287449392715, 8.607287449392715, 8.607287449392715, 7.6072874493927145, 7.6072874493927145, 8.607287449392715, 8.607287449392715, 7.6072874493927145, 7.6072874493927145, 7.6072874493927145, 7.6072874493927145, 7.6072874493927145, 7.6072874493927145, 7.6072874493927145, 7.6072874493927145, 7.6072874493927145, 7.6072874493927145, 7.6072874493927145, 7.6072874493927145, 7.6072874493927145, 7.6072874493927145, 7.6072874493927145, 7.6072874493927145, 7.6072874493927145, 7.6072874493927145, 7.6072874493927145, 7.6072874493927145, 7.6072874493927145, 7.6072874493927145, 7.6072874493927145, 7.6072874493927145, 7.6072874493927145, 7.6072874493927145, 7.6072874493927145, 7.6072874493927145, 7.6072874493927145, 7.6072874493927145, 7.6072874493927145, 7.6072874493927145, 7.6072874493927145, 7.6072874493927145, 7.6072874493927145, 7.6072874493927145, 7.6072874493927145, 7.6072874493927145, 7.6072874493927145, 7.6072874493927145, 7.6072874493927145, 7.6072874493927145, 7.6072874493927145, 7.6072874493927145, 7.6072874493927145, 7.6072874493927145, 7.6072874493927145, 7.6072874493927145, 7.6072874493927145, 7.6072874493927145, 7.6072874493927145, 7.6072874493927145, 7.6072874493927145, 7.6072874493927145, 7.6072874493927145, 7.6072874493927145, 7.6072874493927145, 7.6072874493927145, 7.6072874493927145, 7.6072874493927145, 7.6072874493927145, 7.6072874493927145, 7.6072874493927145, 7.6072874493927145, 7.6072874493927145, 7.6072874493927145, 7.6072874493927145, 7.6072874493927145, 7.6072874493927145, 7.6072874493927145, 7.6072874493927145, 7.6072874493927145, 6.6072874493927145, 7.6072874493927145, 7.6072874493927145, -240.39271255060729, -240.39271255060729, -240.39271255060729, -240.39271255060729, -240.39271255060729, -240.39271255060729, -240.39271255060729, -240.39271255060729, -240.39271255060729, -240.39271255060729, -240.39271255060729, -240.39271255060729, 7.6072874493927145, 7.6072874493927145, 7.6072874493927145, 7.6072874493927145, 7.6072874493927145, 7.6072874493927145, 7.6072874493927145, 7.6072874493927145, 6.6072874493927145, 7.6072874493927145, 7.6072874493927145, 7.6072874493927145, 7.6072874493927145, 6.6072874493927145, 6.6072874493927145, 6.6072874493927145, 7.6072874493927145, 7.6072874493927145, 7.6072874493927145, 7.6072874493927145, 6.6072874493927145, 6.6072874493927145, 7.6072874493927145, 7.6072874493927145, 7.6072874493927145, 7.6072874493927145, 7.6072874493927145, 7.6072874493927145, 7.6072874493927145, 7.6072874493927145, 6.6072874493927145, 6.6072874493927145, 7.6072874493927145, 6.6072874493927145, 7.6072874493927145, 7.6072874493927145, 7.6072874493927145, 6.6072874493927145, 7.6072874493927145, 7.6072874493927145, 7.6072874493927145, 6.6072874493927145, 7.6072874493927145, 7.6072874493927145, 7.6072874493927145, 7.6072874493927145, 7.6072874493927145, 7.6072874493927145, 7.6072874493927145, 7.6072874493927145, 7.6072874493927145, 7.6072874493927145, 7.6072874493927145, 7.6072874493927145, 7.6072874493927145, 7.6072874493927145, 7.6072874493927145, 7.6072874493927145, 7.6072874493927145, 7.6072874493927145, 7.6072874493927145, 7.6072874493927145, 6.6072874493927145, 7.6072874493927145, 7.6072874493927145, 6.6072874493927145, 7.6072874493927145, 7.6072874493927145, 7.6072874493927145, 6.6072874493927145, 7.6072874493927145, 7.6072874493927145, 7.6072874493927145, 6.6072874493927145, 6.6072874493927145, 6.6072874493927145, 6.6072874493927145, 6.6072874493927145, 7.6072874493927145, 7.6072874493927145, 6.6072874493927145, 7.6072874493927145, 6.6072874493927145, 6.6072874493927145, 6.6072874493927145, 6.6072874493927145, 6.6072874493927145, 7.6072874493927145, 6.6072874493927145, 6.6072874493927145, 6.6072874493927145, 7.6072874493927145, 6.6072874493927145, 6.6072874493927145, 6.6072874493927145, 6.6072874493927145, 6.6072874493927145, 6.6072874493927145, 6.6072874493927145, 7.6072874493927145, 6.6072874493927145, 6.6072874493927145, 7.6072874493927145, 6.6072874493927145, 6.6072874493927145, 7.6072874493927145, 7.6072874493927145, 7.6072874493927145, 6.6072874493927145, 7.6072874493927145, 6.6072874493927145, 6.6072874493927145, 6.6072874493927145, 6.6072874493927145, 6.6072874493927145, 6.6072874493927145, 6.6072874493927145, 6.6072874493927145, -0.3927125506072855, 6.6072874493927145, 6.6072874493927145, 6.6072874493927145, 6.6072874493927145, 6.6072874493927145, 6.6072874493927145, 6.6072874493927145, 6.6072874493927145, 6.6072874493927145, 6.6072874493927145, 6.6072874493927145, 6.6072874493927145, 6.6072874493927145, 6.6072874493927145, 6.6072874493927145, 6.6072874493927145, 6.6072874493927145, 6.6072874493927145, 6.6072874493927145, 6.6072874493927145, 6.6072874493927145, 6.6072874493927145, 7.6072874493927145, 6.6072874493927145, 6.6072874493927145, 6.6072874493927145, 6.6072874493927145, 6.6072874493927145, 6.6072874493927145, 6.6072874493927145, 6.6072874493927145, 7.6072874493927145, 6.6072874493927145, 6.6072874493927145, 6.6072874493927145, 6.6072874493927145, 6.6072874493927145, 6.6072874493927145, 6.6072874493927145, 6.6072874493927145, 6.6072874493927145, 6.6072874493927145, 6.6072874493927145, 6.6072874493927145, 6.6072874493927145, 6.6072874493927145, 6.6072874493927145, 6.6072874493927145, 6.6072874493927145, 6.6072874493927145, 6.6072874493927145, 6.6072874493927145, 7.6072874493927145, 6.6072874493927145, 6.6072874493927145, 6.6072874493927145, 6.6072874493927145, 6.6072874493927145, 6.6072874493927145, 6.6072874493927145, 6.6072874493927145, 6.6072874493927145, 6.6072874493927145, 6.6072874493927145, 6.6072874493927145, 6.6072874493927145, 6.6072874493927145, 6.6072874493927145, 6.6072874493927145, 6.6072874493927145, 7.6072874493927145, 6.6072874493927145, 6.6072874493927145, 6.6072874493927145, 7.6072874493927145, 7.6072874493927145, 6.6072874493927145, 6.6072874493927145, 6.6072874493927145, 6.6072874493927145, 6.6072874493927145, 7.6072874493927145, 7.6072874493927145, 6.6072874493927145, 6.6072874493927145, 6.6072874493927145, 6.6072874493927145, 6.6072874493927145, 6.6072874493927145, 6.6072874493927145, 6.6072874493927145, 6.6072874493927145, 6.6072874493927145, 6.6072874493927145, 6.6072874493927145, 6.6072874493927145, 6.6072874493927145, 6.6072874493927145, 6.6072874493927145, 6.6072874493927145, 6.6072874493927145, 6.6072874493927145, 6.6072874493927145, 6.6072874493927145, 6.6072874493927145, 6.6072874493927145, 6.6072874493927145, 6.6072874493927145, 6.6072874493927145, 6.6072874493927145, 6.6072874493927145, 6.6072874493927145, 6.6072874493927145, 6.6072874493927145, 5.6072874493927145, 6.6072874493927145, 6.6072874493927145, 6.6072874493927145, 6.6072874493927145, 6.6072874493927145, 6.6072874493927145, 6.6072874493927145, 6.6072874493927145, 6.6072874493927145, 6.6072874493927145, 6.6072874493927145, 6.6072874493927145, 6.6072874493927145, 6.6072874493927145, 6.6072874493927145, 6.6072874493927145, 6.6072874493927145, 6.6072874493927145, 6.6072874493927145, 6.6072874493927145, 6.6072874493927145, 6.6072874493927145, 6.6072874493927145, 6.6072874493927145, 6.6072874493927145, 6.6072874493927145, 6.6072874493927145, 6.6072874493927145, 6.6072874493927145, 6.6072874493927145, 6.6072874493927145, 6.6072874493927145, 6.6072874493927145, 6.6072874493927145, 6.6072874493927145, 6.6072874493927145, 6.6072874493927145, 6.6072874493927145, 6.6072874493927145, 6.6072874493927145, 6.6072874493927145, 6.6072874493927145, 6.6072874493927145, 6.6072874493927145, 6.6072874493927145, 6.6072874493927145, 6.6072874493927145, 6.6072874493927145, 6.6072874493927145, 6.6072874493927145, 6.6072874493927145, 6.6072874493927145, 6.6072874493927145, 6.6072874493927145, 6.6072874493927145, 6.6072874493927145, 6.6072874493927145, 6.6072874493927145, 6.6072874493927145, 6.6072874493927145, 6.6072874493927145, 6.6072874493927145, 6.6072874493927145, 6.6072874493927145, 6.6072874493927145, 6.6072874493927145, 6.6072874493927145, 6.6072874493927145, 6.6072874493927145, 6.6072874493927145, 6.6072874493927145, 6.6072874493927145, 6.6072874493927145, 6.6072874493927145, 6.6072874493927145, 6.6072874493927145, 6.6072874493927145, 6.6072874493927145, 6.6072874493927145, 6.6072874493927145, 6.6072874493927145, 6.6072874493927145, 6.6072874493927145, 6.6072874493927145, 5.6072874493927145, 6.6072874493927145, 6.6072874493927145, 6.6072874493927145, 6.6072874493927145, 5.6072874493927145, 6.6072874493927145, -0.3927125506072855, 6.6072874493927145, 6.6072874493927145, 6.6072874493927145, 6.6072874493927145, 6.6072874493927145, 6.6072874493927145, 6.6072874493927145, 6.6072874493927145, 6.6072874493927145, 6.6072874493927145, 6.6072874493927145, 6.6072874493927145, 6.6072874493927145, 6.6072874493927145, 6.6072874493927145, 5.6072874493927145, 6.6072874493927145, 6.6072874493927145, 6.6072874493927145, 6.6072874493927145, 6.6072874493927145, 6.6072874493927145, 6.6072874493927145, 6.6072874493927145, 6.6072874493927145, 6.6072874493927145, 6.6072874493927145, 5.6072874493927145, 6.6072874493927145, 6.6072874493927145, 6.6072874493927145, 5.6072874493927145, 5.6072874493927145, 6.6072874493927145, 6.6072874493927145, 6.6072874493927145, 6.6072874493927145, 6.6072874493927145]}]
  out "# of records":i64=495
  out "Array":T1(array[cluster])=[{"Guppy X"=nan, "Guppy Y"=nan, "M3 X"=nan, "M3 Y"=nan, "temp"=2.4800000000000004, "date string"="9/19/2011", "time string"="9:25:59 AM"}, {"Guppy X"=nan, "Guppy Y"=nan, "M3 X"=nan, "M3 Y"=nan, "temp"=0.0, "date string"="9/19/2011", "time string"="9:26:58 AM"}, {"Guppy X"=nan, "Guppy Y"=nan, "M3 X"=nan, "M3 Y"=nan, "temp"=0.0, "date string"="9/19/2011", "time string"="9:28:01 AM"}, {"Guppy X"=nan, "Guppy Y"=nan, "M3 X"=nan, "M3 Y"=nan, "temp"=249.0, "date string"="9/19/2011", "time string"="9:29:01 AM"}, {"Guppy X"=755.1923300170795, "Guppy Y"=684.0665187818796, "M3 X"=405.838373005935, "M3 Y"=324.25062821876577, "temp"=249.0, "date string"="9/19/2011", "time string"="9:30:01 AM"}, {"Guppy X"=755.0917986268107, "Guppy Y"=683.6877666266289, "M3 X"=405.1229625925154, "M3 Y"=324.601335842121, "temp"=249.0, "date string"="9/19/2011", "time string"="9:31:01 AM"}, {"Guppy X"=755.3088452352039, "Guppy Y"=683.503670363707, "M3 X"=404.4959916003411, "M3 Y"=324.32531516008567, "temp"=249.0, "date string"="9/19/2011", "time string"="9:32:08 AM"}, {"Guppy X"=nan, "Guppy Y"=nan, "M3 X"=nan, "M3 Y"=nan, "temp"=249.0, "date string"="9/19/2011", "time string"="9:33:08 AM"}, {"Guppy X"=756.3291937508868, "Guppy Y"=683.7532264415746, "M3 X"=406.2848501971284, "M3 Y"=325.21753593927707, "temp"=249.0, "date string"="9/19/2011", "time string"="9:34:08 AM"}, {"Guppy X"=755.8188140434854, "Guppy Y"=683.4246721072982, "M3 X"=406.772034070845, "M3 Y"=324.9877731475327, "temp"=249.0, "date string"="9/19/2011", "time string"="9:35:08 AM"}, {"Guppy X"=757.1790263711645, "Guppy Y"=683.0602702679753, "M3 X"=408.86161842766137, "M3 Y"=325.3567103571116, "temp"=249.0, "date string"="9/19/2011", "time string"="9:36:08 AM"}, {"Guppy X"=nan, "Guppy Y"=nan, "M3 X"=nan, "M3 Y"=nan, "temp"=248.0, "date string"="9/19/2011", "time string"="9:37:09 AM"}, {"Guppy X"=nan, "Guppy Y"=nan, "M3 X"=nan, "M3 Y"=nan, "temp"=248.0, "date string"="9/19/2011", "time string"="9:38:09 AM"}, {"Guppy X"=756.9120479393266, "Guppy Y"=683.0131512236079, "M3 X"=410.119567234039, "M3 Y"=324.9436386822496, "temp"=248.0, "date string"="9/19/2011", "time string"="9:39:09 AM"}, {"Guppy X"=756.7342802083404, "Guppy Y"=683.8271910907575, "M3 X"=406.2447217205329, "M3 Y"=325.34240001623846, "temp"=248.0, "date string"="9/19/2011", "time string"="9:40:09 AM"}, {"Guppy X"=756.310647368533, "Guppy Y"=684.0962689453371, "M3 X"=407.333369065433, "M3 Y"=325.66755592359993, "temp"=249.0, "date string"="9/19/2011", "time string"="9:41:09 AM"}, {"Guppy X"=756.1189467425046, "Guppy Y"=683.8813470766494, "M3 X"=410.84256663174705, "M3 Y"=325.413803698878, "temp"=249.0, "date string"="9/19/2011", "time string"="9:42:09 AM"}, {"Guppy X"=755.8671078584364, "Guppy Y"=683.8350078463791, "M3 X"=410.719011561617, "M3 Y"=324.40681156495066, "temp"=248.0, "date string"="9/19/2011", "time string"="9:43:10 AM"}, {"Guppy X"=755.7995765148469, "Guppy Y"=684.0297510299794, "M3 X"=409.13963912710375, "M3 Y"=324.6740119230383, "temp"=248.0, "date string"="9/19/2011", "time string"="9:44:10 AM"}, {"Guppy X"=755.443910952569, "Guppy Y"=684.5586357886597, "M3 X"=408.13683408153616, "M3 Y"=324.5788517354078, "temp"=249.0, "date string"="9/19/2011", "time string"="9:45:10 AM"}, {"Guppy X"=755.4285905724633, "Guppy Y"=684.5685798247476, "M3 X"=408.61173228133634, "M3 Y"=324.6787780611582, "temp"=249.0, "date string"="9/19/2011", "time string"="9:46:10 AM"}, {"Guppy X"=755.7851504416609, "Guppy Y"=684.7455640552898, "M3 X"=406.90035727342644, "M3 Y"=324.5471996388034, "temp"=249.0, "date string"="9/19/2011", "time string"="9:47:10 AM"}, {"Guppy X"=756.1377340557982, "Guppy Y"=684.6812069642572, "M3 X"=405.82520763028384, "M3 Y"=324.46425825792153, "temp"=249.0, "date string"="9/19/2011", "time string"="9:48:10 AM"}, {"Guppy X"=754.6067411900464, "Guppy Y"=684.807516860215, "M3 X"=412.41710753415634, "M3 Y"=324.00829853676123, "temp"=248.0, "date string"="9/19/2011", "time string"="9:49:10 AM"}, {"Guppy X"=755.3455928150833, "Guppy Y"=685.0977284992686, "M3 X"=406.3508136501162, "M3 Y"=324.5356710270558, "temp"=249.0, "date string"="9/19/2011", "time string"="9:50:11 AM"}, {"Guppy X"=754.8864748805192, "Guppy Y"=685.1279949836091, "M3 X"=409.4279832336839, "M3 Y"=324.33173575978344, "temp"=248.0, "date string"="9/19/2011", "time string"="9:51:11 AM"}, {"Guppy X"=754.8367080137155, "Guppy Y"=685.38337156947, "M3 X"=407.8482169792964, "M3 Y"=324.6406765340668, "temp"=248.0, "date string"="9/19/2011", "time string"="9:52:11 AM"}, {"Guppy X"=754.9281105525774, "Guppy Y"=685.3947848663345, "M3 X"=409.8053875784576, "M3 Y"=325.80727720115266, "temp"=249.0, "date string"="9/19/2011", "time string"="9:53:11 AM"}, {"Guppy X"=754.3961299925785, "Guppy Y"=685.6475076076015, "M3 X"=408.94038871321834, "M3 Y"=325.4966003176416, "temp"=248.0, "date string"="9/19/2011", "time string"="9:54:11 AM"}, {"Guppy X"=753.6081270799882, "Guppy Y"=685.7474055267772, "M3 X"=411.92743483200735, "M3 Y"=325.3433252503475, "temp"=248.0, "date string"="9/19/2011", "time string"="9:55:11 AM"}, {"Guppy X"=754.3155412788507, "Guppy Y"=685.6888044805579, "M3 X"=410.4262763810612, "M3 Y"=324.92705528198263, "temp"=248.0, "date string"="9/19/2011", "time string"="9:56:11 AM"}, {"Guppy X"=754.0839532069936, "Guppy Y"=685.7353955429886, "M3 X"=409.1695855272571, "M3 Y"=324.90358621083453, "temp"=248.0, "date string"="9/19/2011", "time string"="9:57:11 AM"}, {"Guppy X"=754.1497478694685, "Guppy Y"=685.8176674393193, "M3 X"=410.20033731473893, "M3 Y"=325.96362493234005, "temp"=248.0, "date string"="9/19/2011", "time string"="9:58:11 AM"}, {"Guppy X"=753.5228823866255, "Guppy Y"=686.0036859612758, "M3 X"=411.2233054444954, "M3 Y"=324.6300704511848, "temp"=248.0, "date string"="9/19/2011", "time string"="9:59:12 AM"}, {"Guppy X"=753.7322159369467, "Guppy Y"=685.8383741488685, "M3 X"=410.14213003181356, "M3 Y"=324.6896875171992, "temp"=248.0, "date string"="9/19/2011", "time string"="10:00:12 AM"}, {"Guppy X"=nan, "Guppy Y"=nan, "M3 X"=nan, "M3 Y"=nan, "temp"=248.0, "date string"="9/19/2011", "time string"="10:01:12 AM"}, {"Guppy X"=754.8151567327996, "Guppy Y"=685.6618727108875, "M3 X"=406.0871293272919, "M3 Y"=326.63216597597216, "temp"=249.0, "date string"="9/19/2011", "time string"="10:02:12 AM"}, {"Guppy X"=753.395189204873, "Guppy Y"=686.0327220412588, "M3 X"=409.69613494127924, "M3 Y"=324.23349804370343, "temp"=249.0, "date string"="9/19/2011", "time string"="10:03:12 AM"}, {"Guppy X"=753.5379770923383, "Guppy Y"=685.8951525879148, "M3 X"=408.9207006403462, "M3 Y"=324.69139033142034, "temp"=249.0, "date string"="9/19/2011", "time string"="10:04:12 AM"}, {"Guppy X"=752.8558127228116, "Guppy Y"=686.507018771049, "M3 X"=412.3138693210806, "M3 Y"=324.52135853923903, "temp"=249.0, "date string"="9/19/2011", "time string"="10:05:12 AM"}, {"Guppy X"=753.9531729228341, "Guppy Y"=686.1077966975312, "M3 X"=408.0482231096158, "M3 Y"=325.1848647662053, "temp"=248.0, "date string"="9/19/2011", "time string"="10:06:12 AM"}, {"Guppy X"=753.0114167741001, "Guppy Y"=684.535536931782, "M3 X"=405.86927401639593, "M3 Y"=325.5436641713361, "temp"=248.0, "date string"="9/19/2011", "time string"="10:07:12 AM"}, {"Guppy X"=753.6913488525532, "Guppy Y"=685.9170517600464, "M3 X"=407.2581721498146, "M3 Y"=324.9993724280872, "temp"=249.0, "date string"="9/19/2011", "time string"="10:08:13 AM"}, {"Guppy X"=754.1656760559855, "Guppy Y"=686.3514008266974, "M3 X"=406.1447145682126, "M3 Y"=325.7392758517449, "temp"=249.0, "date string"="9/19/2011", "time string"="10:09:13 AM"}, {"Guppy X"=754.1549676790378, "Guppy Y"=686.3313512261147, "M3 X"=406.1673435871159, "M3 Y"=325.91657315340944, "temp"=248.0, "date string"="9/19/2011", "time string"="10:10:13 AM"}, {"Guppy X"=753.6325792914798, "Guppy Y"=686.5822033445673, "M3 X"=407.22888244618554, "M3 Y"=326.28998490722154, "temp"=248.0, "date string"="9/19/2011", "time string"="10:11:13 AM"}, {"Guppy X"=752.6317165686811, "Guppy Y"=686.9360857591341, "M3 X"=410.3035851834418, "M3 Y"=325.4141256650264, "temp"=248.0, "date string"="9/19/2011", "time string"="10:12:13 AM"}, {"Guppy X"=753.1355859105186, "Guppy Y"=686.6231433787406, "M3 X"=408.38409539059256, "M3 Y"=325.81550361777755, "temp"=248.0, "date string"="9/19/2011", "time string"="10:13:13 AM"}, {"Guppy X"=753.7656949557417, "Guppy Y"=686.4641158787465, "M3 X"=407.0122251051909, "M3 Y"=325.7278088758526, "temp"=248.0, "date string"="9/19/2011", "time string"="10:14:13 AM"}, {"Guppy X"=753.9368068085728, "Guppy Y"=686.3270108184884, "M3 X"=405.5706013496782, "M3 Y"=326.12539074813395, "temp"=248.0, "date string"="9/19/2011", "time string"="10:15:13 AM"}, {"Guppy X"=752.9123162757594, "Guppy Y"=686.843980765385, "M3 X"=409.0303867108499, "M3 Y"=325.7879480424666, "temp"=248.0, "date string"="9/19/2011", "time string"="10:16:13 AM"}, {"Guppy X"=753.7766690119465, "Guppy Y"=686.6374016176122, "M3 X"=406.9734479791718, "M3 Y"=326.2382413034624, "temp"=248.0, "date string"="9/19/2011", "time string"="10:17:13 AM"}, {"Guppy X"=754.0644259199792, "Guppy Y"=686.4123544364178, "M3 X"=405.62844694988087, "M3 Y"=326.58299388985716, "temp"=248.0, "date string"="9/19/2011", "time string"="10:18:13 AM"}, {"Guppy X"=752.7521220577532, "Guppy Y"=685.0855697344807, "M3 X"=405.7029004969868, "M3 Y"=326.0012269387699, "temp"=248.0, "date string"="9/19/2011", "time string"="10:19:13 AM"}, {"Guppy X"=753.308183043187, "Guppy Y"=686.2535126235693, "M3 X"=407.5234147653391, "M3 Y"=324.9022241180587, "temp"=248.0, "date string"="9/19/2011", "time string"="10:20:13 AM"}, {"Guppy X"=755.3517354231057, "Guppy Y"=686.9931515526081, "M3 X"=405.41439447710127, "M3 Y"=327.7156814237586, "temp"=248.0, "date string"="9/19/2011", "time string"="10:21:13 AM"}, {"Guppy X"=754.6762757451527, "Guppy Y"=686.7350368416202, "M3 X"=405.6604641009617, "M3 Y"=327.6555798442115, "temp"=248.0, "date string"="9/19/2011", "time string"="10:22:14 AM"}, {"Guppy X"=755.0669004120558, "Guppy Y"=686.9510454905362, "M3 X"=405.1295511137764, "M3 Y"=327.8830997759124, "temp"=248.0, "date string"="9/19/2011", "time string"="10:23:14 AM"}, {"Guppy X"=755.0294244569336, "Guppy Y"=686.3289510329583, "M3 X"=404.66713372935607, "M3 Y"=327.2049409789625, "temp"=248.0, "date string"="9/19/2011", "time string"="10:24:14 AM"}, {"Guppy X"=754.4992891573185, "Guppy Y"=686.4466091438635, "M3 X"=406.3264309767984, "M3 Y"=328.4107803272773, "temp"=248.0, "date string"="9/19/2011", "time string"="10:25:14 AM"}, {"Guppy X"=754.6774429678887, "Guppy Y"=686.3554031319104, "M3 X"=404.9920432742798, "M3 Y"=327.0132166080609, "temp"=248.0, "date string"="9/19/2011", "time string"="10:26:14 AM"}, {"Guppy X"=754.1303893617824, "Guppy Y"=686.6778470665313, "M3 X"=405.9277808316792, "M3 Y"=326.44500362546023, "temp"=248.0, "date string"="9/19/2011", "time string"="10:27:14 AM"}, {"Guppy X"=754.5446707457534, "Guppy Y"=686.7118612492069, "M3 X"=405.2775712831199, "M3 Y"=326.67158726948196, "temp"=248.0, "date string"="9/19/2011", "time string"="10:28:14 AM"}, {"Guppy X"=754.2299606215458, "Guppy Y"=686.683893236888, "M3 X"=405.67767726489376, "M3 Y"=326.1288912414156, "temp"=248.0, "date string"="9/19/2011", "time string"="10:29:14 AM"}, {"Guppy X"=754.419772233777, "Guppy Y"=686.6704278782279, "M3 X"=405.3804361315767, "M3 Y"=326.5966305801072, "temp"=248.0, "date string"="9/19/2011", "time string"="10:30:15 AM"}, {"Guppy X"=753.7782727814032, "Guppy Y"=686.6077001140394, "M3 X"=405.9853089396176, "M3 Y"=326.87487617317095, "temp"=248.0, "date string"="9/19/2011", "time string"="10:31:15 AM"}, {"Guppy X"=754.7808565293208, "Guppy Y"=686.7732299147344, "M3 X"=404.42672294933254, "M3 Y"=327.5848957206743, "temp"=248.0, "date string"="9/19/2011", "time string"="10:32:15 AM"}, {"Guppy X"=752.7251933063969, "Guppy Y"=687.234557000902, "M3 X"=408.4873939989987, "M3 Y"=325.65466364530454, "temp"=248.0, "date string"="9/19/2011", "time string"="10:33:15 AM"}, {"Guppy X"=754.2644851485795, "Guppy Y"=686.6749073495035, "M3 X"=404.89405030514433, "M3 Y"=326.5234560416922, "temp"=248.0, "date string"="9/19/2011", "time string"="10:34:15 AM"}, {"Guppy X"=754.4231791458328, "Guppy Y"=686.7393062652245, "M3 X"=404.7867412396793, "M3 Y"=326.9088348635029, "temp"=248.0, "date string"="9/19/2011", "time string"="10:35:15 AM"}, {"Guppy X"=748.6547198645156, "Guppy Y"=681.984522358485, "M3 X"=406.33374532263764, "M3 Y"=326.6756532182455, "temp"=248.0, "date string"="9/19/2011", "time string"="10:36:15 AM"}, {"Guppy X"=754.4197793195258, "Guppy Y"=686.9950922966746, "M3 X"=405.0538587868212, "M3 Y"=327.01601856021347, "temp"=248.0, "date string"="9/19/2011", "time string"="10:37:15 AM"}, {"Guppy X"=754.140874533837, "Guppy Y"=687.2025886141937, "M3 X"=405.2959266967243, "M3 Y"=327.15310535573894, "temp"=248.0, "date string"="9/19/2011", "time string"="10:38:16 AM"}, {"Guppy X"=754.471381665849, "Guppy Y"=687.0191834141484, "M3 X"=404.5673526356913, "M3 Y"=326.9034629323913, "temp"=248.0, "date string"="9/19/2011", "time string"="10:39:16 AM"}, {"Guppy X"=754.2157790362683, "Guppy Y"=686.9903027062901, "M3 X"=405.153821563506, "M3 Y"=326.0404548787967, "temp"=248.0, "date string"="9/19/2011", "time string"="10:40:16 AM"}, {"Guppy X"=753.66710949745, "Guppy Y"=687.4001277742107, "M3 X"=405.8481787616453, "M3 Y"=327.0077059432166, "temp"=248.0, "date string"="9/19/2011", "time string"="10:41:16 AM"}, {"Guppy X"=754.347365795313, "Guppy Y"=686.9341934416335, "M3 X"=404.7540578017385, "M3 Y"=326.99871137680304, "temp"=248.0, "date string"="9/19/2011", "time string"="10:42:16 AM"}, {"Guppy X"=753.9967184673219, "Guppy Y"=687.5247541504997, "M3 X"=408.132698272434, "M3 Y"=329.62429596867617, "temp"=248.0, "date string"="9/19/2011", "time string"="10:43:16 AM"}, {"Guppy X"=753.3603791680486, "Guppy Y"=687.738712218767, "M3 X"=406.45607448301865, "M3 Y"=326.04279614038575, "temp"=248.0, "date string"="9/19/2011", "time string"="10:44:16 AM"}, {"Guppy X"=753.5643725689765, "Guppy Y"=687.7826358889507, "M3 X"=405.8355390413879, "M3 Y"=326.68681088887723, "temp"=248.0, "date string"="9/19/2011", "time string"="10:45:16 AM"}, {"Guppy X"=754.6272580922562, "Guppy Y"=687.1576149029751, "M3 X"=404.11796274122275, "M3 Y"=327.41682894311293, "temp"=248.0, "date string"="9/19/2011", "time string"="10:46:16 AM"}, {"Guppy X"=753.8114955266728, "Guppy Y"=687.313055402016, "M3 X"=405.4217429063766, "M3 Y"=326.6053008451733, "temp"=248.0, "date string"="9/19/2011", "time string"="10:47:17 AM"}, {"Guppy X"=754.54100946802, "Guppy Y"=687.0838616654447, "M3 X"=404.077895993349, "M3 Y"=327.1465998362621, "temp"=248.0, "date string"="9/19/2011", "time string"="10:48:17 AM"}, {"Guppy X"=752.5388097637579, "Guppy Y"=687.952583588566, "M3 X"=407.3668063938615, "M3 Y"=325.83681208749596, "temp"=248.0, "date string"="9/19/2011", "time string"="10:49:17 AM"}, {"Guppy X"=753.7971435435667, "Guppy Y"=687.4820749762191, "M3 X"=406.37426887491586, "M3 Y"=327.9293766461715, "temp"=248.0, "date string"="9/19/2011", "time string"="10:50:17 AM"}, {"Guppy X"=753.6163733510139, "Guppy Y"=687.7519171735823, "M3 X"=405.5110271753082, "M3 Y"=326.59945739165227, "temp"=248.0, "date string"="9/19/2011", "time string"="10:51:17 AM"}, {"Guppy X"=752.8752110912297, "Guppy Y"=687.7326990692613, "M3 X"=406.3776410165156, "M3 Y"=326.2513808201278, "temp"=248.0, "date string"="9/19/2011", "time string"="10:52:17 AM"}, {"Guppy X"=752.899154003661, "Guppy Y"=686.2204938801443, "M3 X"=404.0120261023465, "M3 Y"=327.6024918567257, "temp"=248.0, "date string"="9/19/2011", "time string"="10:53:17 AM"}, {"Guppy X"=752.2266462900158, "Guppy Y"=688.0912323136549, "M3 X"=407.11601258777614, "M3 Y"=326.6049609375788, "temp"=248.0, "date string"="9/19/2011", "time string"="10:54:18 AM"}, {"Guppy X"=751.7421165250616, "Guppy Y"=688.284966582713, "M3 X"=408.4559130518149, "M3 Y"=325.01842442669954, "temp"=248.0, "date string"="9/19/2011", "time string"="10:55:18 AM"}, {"Guppy X"=753.440386782499, "Guppy Y"=687.7477383595273, "M3 X"=405.63023045402304, "M3 Y"=326.44910076847765, "temp"=248.0, "date string"="9/19/2011", "time string"="10:56:18 AM"}, {"Guppy X"=753.0135229262356, "Guppy Y"=688.0388723163568, "M3 X"=406.2406512011899, "M3 Y"=326.53254721664837, "temp"=248.0, "date string"="9/19/2011", "time string"="10:57:18 AM"}, {"Guppy X"=750.9934962529135, "Guppy Y"=686.8159285736469, "M3 X"=407.3603275499071, "M3 Y"=325.2246907257797, "temp"=248.0, "date string"="9/19/2011", "time string"="10:58:18 AM"}, {"Guppy X"=754.2951641630573, "Guppy Y"=687.8346537582046, "M3 X"=404.0951030956911, "M3 Y"=327.2875993637965, "temp"=248.0, "date string"="9/19/2011", "time string"="10:59:18 AM"}, {"Guppy X"=753.3727408262218, "Guppy Y"=688.0000022169279, "M3 X"=405.62987058767936, "M3 Y"=326.88965278390697, "temp"=248.0, "date string"="9/19/2011", "time string"="11:00:18 AM"}, {"Guppy X"=753.6254256637328, "Guppy Y"=687.9777557695688, "M3 X"=405.41037635068227, "M3 Y"=326.39869929215865, "temp"=248.0, "date string"="9/19/2011", "time string"="11:01:18 AM"}, {"Guppy X"=753.4295263167219, "Guppy Y"=687.982941936927, "M3 X"=405.47849541280925, "M3 Y"=327.0198458240815, "temp"=248.0, "date string"="9/19/2011", "time string"="11:02:18 AM"}, {"Guppy X"=753.0738790084802, "Guppy Y"=688.0271310806523, "M3 X"=405.3917123930219, "M3 Y"=327.11965221730367, "temp"=248.0, "date string"="9/19/2011", "time string"="11:03:18 AM"}, {"Guppy X"=753.485489817728, "Guppy Y"=688.181385226177, "M3 X"=405.29122406581087, "M3 Y"=326.9536936209836, "temp"=248.0, "date string"="9/19/2011", "time string"="11:04:18 AM"}, {"Guppy X"=751.0852690088911, "Guppy Y"=685.261310888524, "M3 X"=404.94162369673535, "M3 Y"=326.50116749599255, "temp"=248.0, "date string"="9/19/2011", "time string"="11:05:18 AM"}, {"Guppy X"=752.3493200718785, "Guppy Y"=686.8111415677164, "M3 X"=405.1015794498372, "M3 Y"=326.5416162471852, "temp"=248.0, "date string"="9/19/2011", "time string"="11:06:19 AM"}, {"Guppy X"=753.7864790980268, "Guppy Y"=688.0010594060424, "M3 X"=404.699076657354, "M3 Y"=326.9918741356132, "temp"=248.0, "date string"="9/19/2011", "time string"="11:07:19 AM"}, {"Guppy X"=754.2120904080676, "Guppy Y"=687.8808845181269, "M3 X"=404.0275985269285, "M3 Y"=326.12561788711514, "temp"=248.0, "date string"="9/19/2011", "time string"="11:08:19 AM"}, {"Guppy X"=753.6236408828436, "Guppy Y"=688.0841947519207, "M3 X"=404.86906492193435, "M3 Y"=326.6354901081491, "temp"=248.0, "date string"="9/19/2011", "time string"="11:09:19 AM"}, {"Guppy X"=754.0660328232618, "Guppy Y"=688.2993141042072, "M3 X"=404.3449901752349, "M3 Y"=327.2192107178871, "temp"=248.0, "date string"="9/19/2011", "time string"="11:10:19 AM"}, {"Guppy X"=753.273725728541, "Guppy Y"=688.1088665618065, "M3 X"=404.06286127294106, "M3 Y"=326.87373720527467, "temp"=248.0, "date string"="9/19/2011", "time string"="11:11:19 AM"}, {"Guppy X"=752.5893347908107, "Guppy Y"=688.3630203465736, "M3 X"=406.20836438408526, "M3 Y"=326.63553163810604, "temp"=248.0, "date string"="9/19/2011", "time string"="11:12:19 AM"}, {"Guppy X"=753.1164643229943, "Guppy Y"=688.4591738281803, "M3 X"=405.78702323813957, "M3 Y"=326.3670335675116, "temp"=248.0, "date string"="9/19/2011", "time string"="11:13:19 AM"}, {"Guppy X"=753.0944365569503, "Guppy Y"=688.7241895347458, "M3 X"=405.32021181278117, "M3 Y"=326.2725769202796, "temp"=248.0, "date string"="9/19/2011", "time string"="11:14:19 AM"}, {"Guppy X"=754.4463752364551, "Guppy Y"=688.0104340039543, "M3 X"=403.75269539532275, "M3 Y"=326.5358328097848, "temp"=248.0, "date string"="9/19/2011", "time string"="11:15:19 AM"}, {"Guppy X"=753.3197045324906, "Guppy Y"=688.3103884054881, "M3 X"=405.12325659459606, "M3 Y"=326.5183797483985, "temp"=248.0, "date string"="9/19/2011", "time string"="11:16:20 AM"}, {"Guppy X"=753.6755144292646, "Guppy Y"=688.1085092074192, "M3 X"=404.47856471594235, "M3 Y"=326.6870116158036, "temp"=248.0, "date string"="9/19/2011", "time string"="11:17:20 AM"}, {"Guppy X"=753.7930291086876, "Guppy Y"=688.6681765452264, "M3 X"=404.54545597098036, "M3 Y"=327.10419027686646, "temp"=248.0, "date string"="9/19/2011", "time string"="11:18:20 AM"}, {"Guppy X"=753.8424342823157, "Guppy Y"=688.3385473138204, "M3 X"=404.42642406105557, "M3 Y"=326.54253925098845, "temp"=248.0, "date string"="9/19/2011", "time string"="11:19:20 AM"}, {"Guppy X"=753.2401543702711, "Guppy Y"=688.1482351013266, "M3 X"=406.2733102634354, "M3 Y"=327.4963697300257, "temp"=248.0, "date string"="9/19/2011", "time string"="11:20:20 AM"}, {"Guppy X"=751.7996282146372, "Guppy Y"=685.7553072737804, "M3 X"=404.06218718751296, "M3 Y"=327.2428515126248, "temp"=248.0, "date string"="9/19/2011", "time string"="11:21:20 AM"}, {"Guppy X"=754.8092913094789, "Guppy Y"=686.50329129042, "M3 X"=404.03939407882467, "M3 Y"=326.8095365642356, "temp"=247.0, "date string"="9/19/2011", "time string"="11:22:20 AM"}, {"Guppy X"=754.8319811838951, "Guppy Y"=686.4276085879567, "M3 X"=405.13774016104276, "M3 Y"=326.4088528221284, "temp"=248.0, "date string"="9/19/2011", "time string"="11:23:21 AM"}, {"Guppy X"=nan, "Guppy Y"=nan, "M3 X"=404.55044438934243, "M3 Y"=326.34859896004247, "temp"=248.0, "date string"="9/19/2011", "time string"="11:24:20 AM"}, {"Guppy X"=nan, "Guppy Y"=nan, "M3 X"=405.2016653668163, "M3 Y"=325.8487672537243, "temp"=0.0, "date string"="9/19/2011", "time string"="11:25:20 AM"}, {"Guppy X"=nan, "Guppy Y"=nan, "M3 X"=405.32443015622056, "M3 Y"=326.247377004202, "temp"=0.0, "date string"="9/19/2011", "time string"="11:26:21 AM"}, {"Guppy X"=nan, "Guppy Y"=nan, "M3 X"=404.99466542344265, "M3 Y"=326.3382996792584, "temp"=0.0, "date string"="9/19/2011", "time string"="11:27:21 AM"}, {"Guppy X"=nan, "Guppy Y"=nan, "M3 X"=405.095640161688, "M3 Y"=326.0398015616507, "temp"=0.0, "date string"="9/19/2011", "time string"="11:28:21 AM"}, {"Guppy X"=nan, "Guppy Y"=nan, "M3 X"=404.5627074926382, "M3 Y"=325.7956330405892, "temp"=0.0, "date string"="9/19/2011", "time string"="11:29:21 AM"}, {"Guppy X"=nan, "Guppy Y"=nan, "M3 X"=404.9924443931305, "M3 Y"=326.3243532792878, "temp"=0.0, "date string"="9/19/2011", "time string"="11:30:21 AM"}, {"Guppy X"=nan, "Guppy Y"=nan, "M3 X"=404.6553583553861, "M3 Y"=325.9314360227179, "temp"=0.0, "date string"="9/19/2011", "time string"="11:31:21 AM"}, {"Guppy X"=nan, "Guppy Y"=nan, "M3 X"=403.1755203314532, "M3 Y"=326.2777734263793, "temp"=0.0, "date string"="9/19/2011", "time string"="11:32:21 AM"}, {"Guppy X"=nan, "Guppy Y"=nan, "M3 X"=402.68067820275803, "M3 Y"=325.9969787889462, "temp"=0.0, "date string"="9/19/2011", "time string"="11:33:21 AM"}, {"Guppy X"=nan, "Guppy Y"=nan, "M3 X"=405.149211642122, "M3 Y"=325.97823748579316, "temp"=0.0, "date string"="9/19/2011", "time string"="11:34:21 AM"}, {"Guppy X"=nan, "Guppy Y"=nan, "M3 X"=404.7726769787312, "M3 Y"=326.19469349379995, "temp"=0.0, "date string"="9/19/2011", "time string"="11:35:21 AM"}, {"Guppy X"=nan, "Guppy Y"=nan, "M3 X"=405.30809161178945, "M3 Y"=325.74474614557107, "temp"=0.0, "date string"="9/19/2011", "time string"="11:36:21 AM"}, {"Guppy X"=757.1207410333542, "Guppy Y"=686.8324847783158, "M3 X"=403.88555651505305, "M3 Y"=325.9382362614146, "temp"=248.0, "date string"="9/19/2011", "time string"="11:37:21 AM"}, {"Guppy X"=759.9073495157672, "Guppy Y"=687.30146060723, "M3 X"=402.0588444130228, "M3 Y"=326.2294419867711, "temp"=248.0, "date string"="9/19/2011", "time string"="11:38:21 AM"}, {"Guppy X"=759.1886666766562, "Guppy Y"=687.8617578777788, "M3 X"=403.6764625595306, "M3 Y"=326.39423025325317, "temp"=248.0, "date string"="9/19/2011", "time string"="11:39:21 AM"}, {"Guppy X"=758.7163661010958, "Guppy Y"=687.3158903744691, "M3 X"=402.9295318716882, "M3 Y"=325.5410197146102, "temp"=248.0, "date string"="9/19/2011", "time string"="11:40:21 AM"}, {"Guppy X"=756.9700612209991, "Guppy Y"=688.3878463402297, "M3 X"=404.61884870513404, "M3 Y"=327.13689724527035, "temp"=248.0, "date string"="9/19/2011", "time string"="11:41:21 AM"}, {"Guppy X"=756.9198559517228, "Guppy Y"=688.4491178208721, "M3 X"=404.6406224833937, "M3 Y"=326.42850053225243, "temp"=248.0, "date string"="9/19/2011", "time string"="11:42:22 AM"}, {"Guppy X"=756.678928749848, "Guppy Y"=688.2996136301447, "M3 X"=405.06292947508854, "M3 Y"=326.29022232522067, "temp"=248.0, "date string"="9/19/2011", "time string"="11:43:22 AM"}, {"Guppy X"=756.5736186715064, "Guppy Y"=688.0633209649646, "M3 X"=405.0967879023218, "M3 Y"=325.5973844001727, "temp"=248.0, "date string"="9/19/2011", "time string"="11:44:22 AM"}, {"Guppy X"=nan, "Guppy Y"=nan, "M3 X"=nan, "M3 Y"=nan, "temp"=247.0, "date string"="9/19/2011", "time string"="11:45:22 AM"}, {"Guppy X"=756.8108496703809, "Guppy Y"=688.2108168560541, "M3 X"=402.5480877774244, "M3 Y"=325.6434793962355, "temp"=248.0, "date string"="9/19/2011", "time string"="11:46:22 AM"}, {"Guppy X"=756.4757516690111, "Guppy Y"=688.0732128306809, "M3 X"=404.9806954984139, "M3 Y"=325.8744060497107, "temp"=248.0, "date string"="9/19/2011", "time string"="11:47:22 AM"}, {"Guppy X"=753.6550030425692, "Guppy Y"=685.9427885616824, "M3 X"=406.13921594008434, "M3 Y"=325.38026823815517, "temp"=248.0, "date string"="9/19/2011", "time string"="11:48:22 AM"}, {"Guppy X"=756.234205379143, "Guppy Y"=688.5303837991127, "M3 X"=404.93365250505616, "M3 Y"=325.9114544710016, "temp"=248.0, "date string"="9/19/2011", "time string"="11:49:22 AM"}, {"Guppy X"=754.097968076804, "Guppy Y"=688.1727685888048, "M3 X"=405.21925255689393, "M3 Y"=325.69772485360113, "temp"=247.0, "date string"="9/19/2011", "time string"="11:50:23 AM"}, {"Guppy X"=753.9223954895577, "Guppy Y"=687.1746771395981, "M3 X"=405.65196560886073, "M3 Y"=324.88667913163664, "temp"=247.0, "date string"="9/19/2011", "time string"="11:51:23 AM"}, {"Guppy X"=753.9570882801142, "Guppy Y"=688.2039203149216, "M3 X"=404.4620216372933, "M3 Y"=325.1569921220712, "temp"=247.0, "date string"="9/19/2011", "time string"="11:52:23 AM"}, {"Guppy X"=753.724518201321, "Guppy Y"=688.2186471865156, "M3 X"=404.9073885245762, "M3 Y"=325.5123004400994, "temp"=248.0, "date string"="9/19/2011", "time string"="11:53:23 AM"}, {"Guppy X"=753.3742215394559, "Guppy Y"=688.3180492151397, "M3 X"=405.2234311401724, "M3 Y"=325.63453823365626, "temp"=248.0, "date string"="9/19/2011", "time string"="11:54:23 AM"}, {"Guppy X"=753.6524118029581, "Guppy Y"=688.461975329057, "M3 X"=404.50610803025216, "M3 Y"=325.44359078558347, "temp"=248.0, "date string"="9/19/2011", "time string"="11:55:23 AM"}, {"Guppy X"=753.5606908680631, "Guppy Y"=688.4954689289958, "M3 X"=404.9864354628487, "M3 Y"=325.04050064497414, "temp"=248.0, "date string"="9/19/2011", "time string"="11:56:23 AM"}, {"Guppy X"=753.3917717420786, "Guppy Y"=688.5637610835305, "M3 X"=405.1725463143489, "M3 Y"=325.07158710840463, "temp"=247.0, "date string"="9/19/2011", "time string"="11:57:23 AM"}, {"Guppy X"=753.2114398944285, "Guppy Y"=688.3951087852296, "M3 X"=405.22473465606174, "M3 Y"=324.8576981104086, "temp"=247.0, "date string"="9/19/2011", "time string"="11:58:23 AM"}, {"Guppy X"=753.2416558992951, "Guppy Y"=688.3738806453648, "M3 X"=405.27904176462914, "M3 Y"=324.9480572448017, "temp"=248.0, "date string"="9/19/2011", "time string"="11:59:23 AM"}, {"Guppy X"=753.5637571924017, "Guppy Y"=688.8221314991179, "M3 X"=403.940708228295, "M3 Y"=325.67844188557785, "temp"=248.0, "date string"="9/19/2011", "time string"="12:00:24 PM"}, {"Guppy X"=753.8264712663248, "Guppy Y"=688.5466740504962, "M3 X"=404.3129761324256, "M3 Y"=324.94542889863885, "temp"=248.0, "date string"="9/19/2011", "time string"="12:01:24 PM"}, {"Guppy X"=753.2625459518155, "Guppy Y"=688.8075214436813, "M3 X"=405.19114235925366, "M3 Y"=325.27848526197783, "temp"=248.0, "date string"="9/19/2011", "time string"="12:02:24 PM"}, {"Guppy X"=753.6236609949649, "Guppy Y"=689.0418420016211, "M3 X"=404.8194039560119, "M3 Y"=325.3928133639521, "temp"=248.0, "date string"="9/19/2011", "time string"="12:03:24 PM"}, {"Guppy X"=748.4954673218286, "Guppy Y"=683.9484880878587, "M3 X"=404.9713106329503, "M3 Y"=325.2087463429589, "temp"=248.0, "date string"="9/19/2011", "time string"="12:04:24 PM"}, {"Guppy X"=752.8132522593113, "Guppy Y"=688.9471123800125, "M3 X"=405.06582011308, "M3 Y"=324.9174121273132, "temp"=248.0, "date string"="9/19/2011", "time string"="12:05:24 PM"}, {"Guppy X"=753.0558642591379, "Guppy Y"=688.894829681566, "M3 X"=405.63109710065413, "M3 Y"=326.37303741548794, "temp"=248.0, "date string"="9/19/2011", "time string"="12:06:24 PM"}, {"Guppy X"=752.7827481938143, "Guppy Y"=689.0166139800389, "M3 X"=405.55412621224764, "M3 Y"=325.2439595173542, "temp"=247.0, "date string"="9/19/2011", "time string"="12:07:24 PM"}, {"Guppy X"=753.2617278195406, "Guppy Y"=688.8990813208193, "M3 X"=405.09966288010287, "M3 Y"=325.0178284003731, "temp"=247.0, "date string"="9/19/2011", "time string"="12:08:24 PM"}, {"Guppy X"=749.9475176727303, "Guppy Y"=685.4029348183496, "M3 X"=404.2951034283975, "M3 Y"=325.55095960433937, "temp"=248.0, "date string"="9/19/2011", "time string"="12:09:25 PM"}, {"Guppy X"=752.9136751168728, "Guppy Y"=689.1344714462047, "M3 X"=404.9526218099542, "M3 Y"=325.63229500209115, "temp"=247.0, "date string"="9/19/2011", "time string"="12:10:25 PM"}, {"Guppy X"=751.1159133664628, "Guppy Y"=686.7481707236556, "M3 X"=405.13594142377207, "M3 Y"=325.0754208729575, "temp"=248.0, "date string"="9/19/2011", "time string"="12:11:25 PM"}, {"Guppy X"=752.6739838254831, "Guppy Y"=689.3218791829963, "M3 X"=406.3302992563571, "M3 Y"=325.15389967744886, "temp"=248.0, "date string"="9/19/2011", "time string"="12:12:25 PM"}, {"Guppy X"=752.9772009581295, "Guppy Y"=689.2494243544136, "M3 X"=405.24390170494127, "M3 Y"=324.8140622683916, "temp"=248.0, "date string"="9/19/2011", "time string"="12:13:25 PM"}, {"Guppy X"=752.457851914264, "Guppy Y"=689.5422739441887, "M3 X"=405.26780788576906, "M3 Y"=324.62915827205353, "temp"=247.0, "date string"="9/19/2011", "time string"="12:14:25 PM"}, {"Guppy X"=753.1482489693626, "Guppy Y"=689.4095924077086, "M3 X"=404.90898555932114, "M3 Y"=324.355919963133, "temp"=248.0, "date string"="9/19/2011", "time string"="12:15:25 PM"}, {"Guppy X"=753.2628243328298, "Guppy Y"=689.5707415510152, "M3 X"=404.6804288117557, "M3 Y"=324.86172616050766, "temp"=248.0, "date string"="9/19/2011", "time string"="12:16:25 PM"}, {"Guppy X"=752.779838706685, "Guppy Y"=689.3969024147187, "M3 X"=407.0257253501733, "M3 Y"=325.44270002409365, "temp"=248.0, "date string"="9/19/2011", "time string"="12:17:25 PM"}, {"Guppy X"=752.6289971413282, "Guppy Y"=689.4735501547167, "M3 X"=405.37785473183766, "M3 Y"=324.6074519778652, "temp"=247.0, "date string"="9/19/2011", "time string"="12:18:26 PM"}, {"Guppy X"=752.6447478818999, "Guppy Y"=689.6357470329502, "M3 X"=405.4821570762373, "M3 Y"=324.75240236829154, "temp"=248.0, "date string"="9/19/2011", "time string"="12:19:26 PM"}, {"Guppy X"=752.3860109901774, "Guppy Y"=689.5838441739577, "M3 X"=405.73388333144925, "M3 Y"=324.7226915005796, "temp"=248.0, "date string"="9/19/2011", "time string"="12:20:26 PM"}, {"Guppy X"=752.7594636610932, "Guppy Y"=689.3010918732032, "M3 X"=405.596564721787, "M3 Y"=325.22428687639194, "temp"=248.0, "date string"="9/19/2011", "time string"="12:21:26 PM"}, {"Guppy X"=752.9830197795744, "Guppy Y"=689.6487738224251, "M3 X"=404.9766628728673, "M3 Y"=325.6501522983824, "temp"=248.0, "date string"="9/19/2011", "time string"="12:22:26 PM"}, {"Guppy X"=752.2758933480649, "Guppy Y"=689.7278521796088, "M3 X"=405.285608725421, "M3 Y"=324.93862484623094, "temp"=248.0, "date string"="9/19/2011", "time string"="12:23:26 PM"}, {"Guppy X"=752.0387360840947, "Guppy Y"=689.9219649770156, "M3 X"=408.11854244943675, "M3 Y"=327.7869277876167, "temp"=248.0, "date string"="9/19/2011", "time string"="12:24:26 PM"}, {"Guppy X"=751.678064641444, "Guppy Y"=689.9401411049881, "M3 X"=405.12899134211716, "M3 Y"=324.7899252010738, "temp"=248.0, "date string"="9/19/2011", "time string"="12:25:26 PM"}, {"Guppy X"=749.0869744226685, "Guppy Y"=686.0684858372308, "M3 X"=406.29189004381846, "M3 Y"=325.49478773931315, "temp"=248.0, "date string"="9/19/2011", "time string"="12:26:26 PM"}, {"Guppy X"=752.6198593334726, "Guppy Y"=690.037571800517, "M3 X"=404.98784817493083, "M3 Y"=325.3180320242787, "temp"=248.0, "date string"="9/19/2011", "time string"="12:27:26 PM"}, {"Guppy X"=752.4464221009578, "Guppy Y"=689.8225444413954, "M3 X"=406.06743088376635, "M3 Y"=324.5203773388565, "temp"=248.0, "date string"="9/19/2011", "time string"="12:28:26 PM"}, {"Guppy X"=752.9366348197847, "Guppy Y"=689.9559903060322, "M3 X"=405.5967996505179, "M3 Y"=325.23641327311987, "temp"=248.0, "date string"="9/19/2011", "time string"="12:29:27 PM"}, {"Guppy X"=752.4097469176728, "Guppy Y"=689.7304456839057, "M3 X"=406.35831320585265, "M3 Y"=325.2542825788169, "temp"=248.0, "date string"="9/19/2011", "time string"="12:30:27 PM"}, {"Guppy X"=752.3933867509674, "Guppy Y"=689.6889402341781, "M3 X"=405.7323447466548, "M3 Y"=324.719600324326, "temp"=248.0, "date string"="9/19/2011", "time string"="12:31:27 PM"}, {"Guppy X"=752.0349475381536, "Guppy Y"=689.8405387668195, "M3 X"=406.0783158674204, "M3 Y"=324.4121420602184, "temp"=248.0, "date string"="9/19/2011", "time string"="12:32:27 PM"}, {"Guppy X"=751.7204945367118, "Guppy Y"=689.9405860091076, "M3 X"=406.25743901567915, "M3 Y"=324.3494140184475, "temp"=248.0, "date string"="9/19/2011", "time string"="12:33:27 PM"}, {"Guppy X"=752.3981310791983, "Guppy Y"=689.8481672358012, "M3 X"=406.46073865464297, "M3 Y"=324.4961063378178, "temp"=248.0, "date string"="9/19/2011", "time string"="12:34:27 PM"}, {"Guppy X"=751.7746320754312, "Guppy Y"=690.1146092883461, "M3 X"=407.4692176243733, "M3 Y"=325.8891787714672, "temp"=248.0, "date string"="9/19/2011", "time string"="12:35:27 PM"}, {"Guppy X"=751.9558641999448, "Guppy Y"=690.2876587475603, "M3 X"=406.3607150124934, "M3 Y"=324.6049999511436, "temp"=248.0, "date string"="9/19/2011", "time string"="12:36:27 PM"}, {"Guppy X"=751.9083724435525, "Guppy Y"=690.1146780682722, "M3 X"=406.19544702920115, "M3 Y"=324.413949144424, "temp"=248.0, "date string"="9/19/2011", "time string"="12:37:27 PM"}, {"Guppy X"=752.5731661883954, "Guppy Y"=690.1560418481911, "M3 X"=406.3046877432004, "M3 Y"=324.9023861835737, "temp"=248.0, "date string"="9/19/2011", "time string"="12:38:28 PM"}, {"Guppy X"=752.5559320689101, "Guppy Y"=690.1797678840613, "M3 X"=404.85812527803756, "M3 Y"=325.1438102770088, "temp"=247.0, "date string"="9/19/2011", "time string"="12:39:28 PM"}, {"Guppy X"=752.7026026414765, "Guppy Y"=690.1887297914825, "M3 X"=405.57346630500854, "M3 Y"=324.6412911704844, "temp"=248.0, "date string"="9/19/2011", "time string"="12:40:28 PM"}, {"Guppy X"=752.6231162162087, "Guppy Y"=690.227979841198, "M3 X"=406.35527977766355, "M3 Y"=324.94509425591787, "temp"=248.0, "date string"="9/19/2011", "time string"="12:41:28 PM"}, {"Guppy X"=751.2389231039964, "Guppy Y"=688.8292740358232, "M3 X"=405.93766885147903, "M3 Y"=326.0940647144592, "temp"=247.0, "date string"="9/19/2011", "time string"="12:42:28 PM"}, {"Guppy X"=752.0154885725319, "Guppy Y"=690.1936691921578, "M3 X"=407.11541897852044, "M3 Y"=324.6986151611766, "temp"=248.0, "date string"="9/19/2011", "time string"="12:43:28 PM"}, {"Guppy X"=752.1325459873791, "Guppy Y"=690.2814806614931, "M3 X"=406.90168398579976, "M3 Y"=324.695775604815, "temp"=248.0, "date string"="9/19/2011", "time string"="12:44:28 PM"}, {"Guppy X"=750.801603464714, "Guppy Y"=688.9255379089414, "M3 X"=406.498390921819, "M3 Y"=324.3962318545673, "temp"=248.0, "date string"="9/19/2011", "time string"="12:45:28 PM"}, {"Guppy X"=752.7105192764152, "Guppy Y"=690.0123160753329, "M3 X"=402.80569705099276, "M3 Y"=324.68637708196076, "temp"=247.0, "date string"="9/19/2011", "time string"="12:46:28 PM"}, {"Guppy X"=752.0692832230986, "Guppy Y"=690.3269068790627, "M3 X"=405.7767272257057, "M3 Y"=324.3914076304662, "temp"=248.0, "date string"="9/19/2011", "time string"="12:47:29 PM"}, {"Guppy X"=752.2685358834837, "Guppy Y"=690.4179408021715, "M3 X"=404.8771549791615, "M3 Y"=324.4751329318429, "temp"=248.0, "date string"="9/19/2011", "time string"="12:48:29 PM"}, {"Guppy X"=751.9087256832731, "Guppy Y"=690.2700672763303, "M3 X"=407.6145030246632, "M3 Y"=324.2569208402824, "temp"=248.0, "date string"="9/19/2011", "time string"="12:49:29 PM"}, {"Guppy X"=752.6349268569633, "Guppy Y"=690.3802087821734, "M3 X"=406.57255648345, "M3 Y"=324.5719687914149, "temp"=247.0, "date string"="9/19/2011", "time string"="12:50:29 PM"}, {"Guppy X"=751.8289457765944, "Guppy Y"=690.4494397938473, "M3 X"=406.999766425766, "M3 Y"=324.04789555531175, "temp"=247.0, "date string"="9/19/2011", "time string"="12:51:29 PM"}, {"Guppy X"=751.8527968512113, "Guppy Y"=690.4176261694461, "M3 X"=407.3638561801222, "M3 Y"=323.9458331101028, "temp"=247.0, "date string"="9/19/2011", "time string"="12:52:29 PM"}, {"Guppy X"=752.2059815285363, "Guppy Y"=690.6942222429627, "M3 X"=406.8079547040477, "M3 Y"=324.36202435428817, "temp"=247.0, "date string"="9/19/2011", "time string"="12:53:29 PM"}, {"Guppy X"=751.6569590465523, "Guppy Y"=690.5885314806152, "M3 X"=406.46798894878776, "M3 Y"=324.0505483469977, "temp"=247.0, "date string"="9/19/2011", "time string"="12:54:29 PM"}, {"Guppy X"=751.5835722655304, "Guppy Y"=690.5329361456127, "M3 X"=406.94286601725355, "M3 Y"=324.0167836608834, "temp"=248.0, "date string"="9/19/2011", "time string"="12:55:29 PM"}, {"Guppy X"=751.4239801093746, "Guppy Y"=690.5161885770908, "M3 X"=406.75446430327116, "M3 Y"=323.16440920609404, "temp"=248.0, "date string"="9/19/2011", "time string"="12:56:29 PM"}, {"Guppy X"=751.6306548757191, "Guppy Y"=690.9121522656058, "M3 X"=406.7584341468057, "M3 Y"=324.07797307642414, "temp"=247.0, "date string"="9/19/2011", "time string"="12:57:29 PM"}, {"Guppy X"=751.5134879539653, "Guppy Y"=690.727041011608, "M3 X"=406.3939220498491, "M3 Y"=323.9405544032073, "temp"=248.0, "date string"="9/19/2011", "time string"="12:58:30 PM"}, {"Guppy X"=751.9465859372034, "Guppy Y"=690.5480388879257, "M3 X"=406.60424479710684, "M3 Y"=323.8333890356494, "temp"=247.0, "date string"="9/19/2011", "time string"="12:59:30 PM"}, {"Guppy X"=750.2624241805894, "Guppy Y"=689.4766075943454, "M3 X"=407.0418976452521, "M3 Y"=323.97149127654814, "temp"=247.0, "date string"="9/19/2011", "time string"="1:00:30 PM"}, {"Guppy X"=749.3985175965303, "Guppy Y"=688.2687462572279, "M3 X"=407.16985729037344, "M3 Y"=323.67246845411495, "temp"=247.0, "date string"="9/19/2011", "time string"="1:01:30 PM"}, {"Guppy X"=750.3069800982743, "Guppy Y"=689.4077081291639, "M3 X"=406.73773728428995, "M3 Y"=323.4432824342906, "temp"=247.0, "date string"="9/19/2011", "time string"="1:02:30 PM"}, {"Guppy X"=751.2535032050868, "Guppy Y"=689.2308884313813, "M3 X"=404.1407563708877, "M3 Y"=323.8282594271612, "temp"=247.0, "date string"="9/19/2011", "time string"="1:03:30 PM"}, {"Guppy X"=752.3979464063799, "Guppy Y"=690.4565081113693, "M3 X"=403.9221909690363, "M3 Y"=323.5828298866705, "temp"=248.0, "date string"="9/19/2011", "time string"="1:04:30 PM"}, {"Guppy X"=752.3059723480916, "Guppy Y"=690.8999040273205, "M3 X"=406.59377061999743, "M3 Y"=323.7566958260285, "temp"=247.0, "date string"="9/19/2011", "time string"="1:05:30 PM"}, {"Guppy X"=751.7573367894797, "Guppy Y"=690.7321137791309, "M3 X"=406.8855523095337, "M3 Y"=322.9845799717199, "temp"=247.0, "date string"="9/19/2011", "time string"="1:06:31 PM"}, {"Guppy X"=751.0858897177111, "Guppy Y"=691.0830964488227, "M3 X"=407.4991170684362, "M3 Y"=322.95213458405414, "temp"=247.0, "date string"="9/19/2011", "time string"="1:07:31 PM"}, {"Guppy X"=751.2454517284875, "Guppy Y"=690.8597496888539, "M3 X"=407.84231302894574, "M3 Y"=322.7437972681998, "temp"=248.0, "date string"="9/19/2011", "time string"="1:08:31 PM"}, {"Guppy X"=751.1143538085231, "Guppy Y"=690.8049082902154, "M3 X"=407.5164783493946, "M3 Y"=322.9802725508218, "temp"=247.0, "date string"="9/19/2011", "time string"="1:09:31 PM"}, {"Guppy X"=751.4106205372806, "Guppy Y"=690.9096514404632, "M3 X"=407.79733986794315, "M3 Y"=323.446505261989, "temp"=247.0, "date string"="9/19/2011", "time string"="1:10:31 PM"}, {"Guppy X"=751.7677490162581, "Guppy Y"=690.9922846075322, "M3 X"=407.79490310362195, "M3 Y"=323.3966561805521, "temp"=247.0, "date string"="9/19/2011", "time string"="1:11:31 PM"}, {"Guppy X"=751.6690491802586, "Guppy Y"=691.117201166387, "M3 X"=407.3494156610997, "M3 Y"=322.98755857290644, "temp"=247.0, "date string"="9/19/2011", "time string"="1:12:31 PM"}, {"Guppy X"=750.9051932142564, "Guppy Y"=691.076462222309, "M3 X"=407.2011646790969, "M3 Y"=322.36761397396344, "temp"=247.0, "date string"="9/19/2011", "time string"="1:13:31 PM"}, {"Guppy X"=751.5623436169545, "Guppy Y"=691.1615557795576, "M3 X"=408.8358862520566, "M3 Y"=324.5642152252239, "temp"=247.0, "date string"="9/19/2011", "time string"="1:14:31 PM"}, {"Guppy X"=751.5837721262251, "Guppy Y"=690.8216369568478, "M3 X"=409.2702729440382, "M3 Y"=324.0666410046724, "temp"=247.0, "date string"="9/19/2011", "time string"="1:15:31 PM"}, {"Guppy X"=751.7695935278801, "Guppy Y"=690.9948845476922, "M3 X"=408.021144094049, "M3 Y"=322.8020173430575, "temp"=248.0, "date string"="9/19/2011", "time string"="1:16:32 PM"}, {"Guppy X"=750.7036850043861, "Guppy Y"=691.2615784970706, "M3 X"=407.3170437508266, "M3 Y"=322.89425453536455, "temp"=247.0, "date string"="9/19/2011", "time string"="1:17:32 PM"}, {"Guppy X"=751.6338230316354, "Guppy Y"=691.3805032407147, "M3 X"=409.4636256972881, "M3 Y"=324.79758792286634, "temp"=247.0, "date string"="9/19/2011", "time string"="1:18:32 PM"}, {"Guppy X"=751.7172200491581, "Guppy Y"=691.1369059306612, "M3 X"=407.64785008363606, "M3 Y"=322.98089325727074, "temp"=248.0, "date string"="9/19/2011", "time string"="1:19:32 PM"}, {"Guppy X"=752.135425872123, "Guppy Y"=691.0591268997642, "M3 X"=407.6414213567256, "M3 Y"=323.8605698163633, "temp"=247.0, "date string"="9/19/2011", "time string"="1:20:32 PM"}, {"Guppy X"=751.2124915598542, "Guppy Y"=691.3065371334271, "M3 X"=408.6781436144292, "M3 Y"=323.0823672811472, "temp"=247.0, "date string"="9/19/2011", "time string"="1:21:32 PM"}, {"Guppy X"=750.7804866219283, "Guppy Y"=691.3332949356878, "M3 X"=408.09886140912664, "M3 Y"=322.7542150871271, "temp"=248.0, "date string"="9/19/2011", "time string"="1:22:32 PM"}, {"Guppy X"=751.3580680733882, "Guppy Y"=691.380271028314, "M3 X"=408.2113129348024, "M3 Y"=322.82221274056855, "temp"=248.0, "date string"="9/19/2011", "time string"="1:23:33 PM"}, {"Guppy X"=750.7535269642203, "Guppy Y"=691.3511490295489, "M3 X"=409.439975564735, "M3 Y"=324.0514158847851, "temp"=248.0, "date string"="9/19/2011", "time string"="1:24:32 PM"}, {"Guppy X"=751.254298625954, "Guppy Y"=691.2441955870055, "M3 X"=407.88981599225343, "M3 Y"=322.98446232262137, "temp"=247.0, "date string"="9/19/2011", "time string"="1:25:33 PM"}, {"Guppy X"=751.6494810208798, "Guppy Y"=691.4737460165992, "M3 X"=408.6172905503616, "M3 Y"=324.71105773744927, "temp"=248.0, "date string"="9/19/2011", "time string"="1:26:33 PM"}, {"Guppy X"=751.5690857089759, "Guppy Y"=691.4478103466797, "M3 X"=408.92164802082704, "M3 Y"=324.35469168141157, "temp"=247.0, "date string"="9/19/2011", "time string"="1:27:33 PM"}, {"Guppy X"=751.1414723116029, "Guppy Y"=691.3796287445018, "M3 X"=408.43933316425836, "M3 Y"=323.2669421346493, "temp"=247.0, "date string"="9/19/2011", "time string"="1:28:33 PM"}, {"Guppy X"=751.4554768537527, "Guppy Y"=691.1097393059873, "M3 X"=406.60614010505515, "M3 Y"=323.5953142804392, "temp"=247.0, "date string"="9/19/2011", "time string"="1:29:33 PM"}, {"Guppy X"=751.476733644965, "Guppy Y"=691.5804933833649, "M3 X"=408.46659841283906, "M3 Y"=323.6293020568495, "temp"=247.0, "date string"="9/19/2011", "time string"="1:30:33 PM"}, {"Guppy X"=749.1463799471578, "Guppy Y"=688.943231684454, "M3 X"=408.39636887605917, "M3 Y"=323.4578847422021, "temp"=247.0, "date string"="9/19/2011", "time string"="1:31:33 PM"}, {"Guppy X"=751.2477607987629, "Guppy Y"=691.46980572295, "M3 X"=408.9335144902082, "M3 Y"=322.72582790515656, "temp"=247.0, "date string"="9/19/2011", "time string"="1:32:34 PM"}, {"Guppy X"=751.7025435621723, "Guppy Y"=691.7078937284853, "M3 X"=407.8432078071359, "M3 Y"=322.6506992386401, "temp"=247.0, "date string"="9/19/2011", "time string"="1:33:34 PM"}, {"Guppy X"=751.664561168508, "Guppy Y"=691.3005879670047, "M3 X"=405.8409437250794, "M3 Y"=324.3308897353647, "temp"=247.0, "date string"="9/19/2011", "time string"="1:34:34 PM"}, {"Guppy X"=751.6165886530872, "Guppy Y"=691.9925894584829, "M3 X"=408.52494146446094, "M3 Y"=323.09821307744863, "temp"=240.0, "date string"="9/19/2011", "time string"="1:35:34 PM"}, {"Guppy X"=751.2388273539201, "Guppy Y"=691.723417558803, "M3 X"=409.0945326721004, "M3 Y"=322.70869171787285, "temp"=247.0, "date string"="9/19/2011", "time string"="1:36:34 PM"}, {"Guppy X"=751.1536584925577, "Guppy Y"=691.4479837193228, "M3 X"=408.52243530671126, "M3 Y"=321.95035019242465, "temp"=247.0, "date string"="9/19/2011", "time string"="1:37:34 PM"}, {"Guppy X"=750.3121256235278, "Guppy Y"=691.7678597518204, "M3 X"=409.2481713967952, "M3 Y"=322.0548786284315, "temp"=247.0, "date string"="9/19/2011", "time string"="1:38:34 PM"}, {"Guppy X"=750.1422580897079, "Guppy Y"=691.7351750321873, "M3 X"=409.1960362379643, "M3 Y"=322.60221242139784, "temp"=247.0, "date string"="9/19/2011", "time string"="1:39:34 PM"}, {"Guppy X"=751.0218329719281, "Guppy Y"=691.7026375434976, "M3 X"=409.21683880194183, "M3 Y"=322.7268172893741, "temp"=247.0, "date string"="9/19/2011", "time string"="1:40:34 PM"}, {"Guppy X"=751.2363142585089, "Guppy Y"=691.6089463940045, "M3 X"=408.56908129637196, "M3 Y"=322.96601016027495, "temp"=247.0, "date string"="9/19/2011", "time string"="1:41:35 PM"}, {"Guppy X"=751.4512311575214, "Guppy Y"=691.7180362982914, "M3 X"=409.6193470388462, "M3 Y"=324.13038549845055, "temp"=247.0, "date string"="9/19/2011", "time string"="1:42:35 PM"}, {"Guppy X"=750.9108892668852, "Guppy Y"=691.8401094655387, "M3 X"=410.67749764232485, "M3 Y"=323.70933337810413, "temp"=247.0, "date string"="9/19/2011", "time string"="1:43:35 PM"}, {"Guppy X"=751.4385119221848, "Guppy Y"=691.8397142708618, "M3 X"=407.98927114812864, "M3 Y"=323.17316525920074, "temp"=247.0, "date string"="9/19/2011", "time string"="1:44:35 PM"}, {"Guppy X"=751.8850873178895, "Guppy Y"=691.9818727458047, "M3 X"=408.2581891526677, "M3 Y"=323.50031075349665, "temp"=247.0, "date string"="9/19/2011", "time string"="1:45:35 PM"}, {"Guppy X"=751.2294422402614, "Guppy Y"=691.993840877182, "M3 X"=409.28095471139335, "M3 Y"=325.3558668127286, "temp"=247.0, "date string"="9/19/2011", "time string"="1:46:35 PM"}, {"Guppy X"=751.8618506175856, "Guppy Y"=691.957183060839, "M3 X"=409.1908083586362, "M3 Y"=326.5450582087532, "temp"=247.0, "date string"="9/19/2011", "time string"="1:47:35 PM"}, {"Guppy X"=752.7521021194934, "Guppy Y"=691.8023707230576, "M3 X"=409.14082729592354, "M3 Y"=324.0257335990222, "temp"=247.0, "date string"="9/19/2011", "time string"="1:48:35 PM"}, {"Guppy X"=752.6208534886189, "Guppy Y"=691.8801359954084, "M3 X"=409.13085023514407, "M3 Y"=322.9217345080266, "temp"=247.0, "date string"="9/19/2011", "time string"="1:49:35 PM"}, {"Guppy X"=749.9157500018815, "Guppy Y"=689.31923595648, "M3 X"=409.9194548193404, "M3 Y"=321.662862210307, "temp"=247.0, "date string"="9/19/2011", "time string"="1:50:35 PM"}, {"Guppy X"=752.5870735586407, "Guppy Y"=691.83095774038, "M3 X"=409.4718435958123, "M3 Y"=321.4360601782811, "temp"=247.0, "date string"="9/19/2011", "time string"="1:51:35 PM"}, {"Guppy X"=752.0467549854645, "Guppy Y"=691.8748492204685, "M3 X"=410.26964290889305, "M3 Y"=321.16016393473654, "temp"=247.0, "date string"="9/19/2011", "time string"="1:52:36 PM"}, {"Guppy X"=751.7699745882492, "Guppy Y"=691.8071414320947, "M3 X"=409.69451092063247, "M3 Y"=321.5908378970846, "temp"=247.0, "date string"="9/19/2011", "time string"="1:53:36 PM"}, {"Guppy X"=749.8944500429578, "Guppy Y"=689.4855213483081, "M3 X"=409.80501148024473, "M3 Y"=321.8680003352, "temp"=247.0, "date string"="9/19/2011", "time string"="1:54:36 PM"}, {"Guppy X"=752.62825846277, "Guppy Y"=692.0344932484652, "M3 X"=409.3616511880555, "M3 Y"=321.8635435630803, "temp"=247.0, "date string"="9/19/2011", "time string"="1:55:36 PM"}, {"Guppy X"=752.0302771295799, "Guppy Y"=691.9776359410544, "M3 X"=409.98709754449607, "M3 Y"=321.5380446305915, "temp"=247.0, "date string"="9/19/2011", "time string"="1:56:36 PM"}, {"Guppy X"=753.0618243746517, "Guppy Y"=691.6777756558005, "M3 X"=406.8252972821278, "M3 Y"=321.44946947254823, "temp"=247.0, "date string"="9/19/2011", "time string"="1:57:36 PM"}, {"Guppy X"=752.5617573780343, "Guppy Y"=691.933134813412, "M3 X"=408.6796165456303, "M3 Y"=321.5252767563623, "temp"=248.0, "date string"="9/19/2011", "time string"="1:58:36 PM"}, {"Guppy X"=752.3519389234053, "Guppy Y"=691.9838851694309, "M3 X"=409.61943219362354, "M3 Y"=321.210709762177, "temp"=247.0, "date string"="9/19/2011", "time string"="1:59:36 PM"}, {"Guppy X"=752.1317059499194, "Guppy Y"=692.0003991815651, "M3 X"=409.53942192987705, "M3 Y"=322.5120230968862, "temp"=247.0, "date string"="9/19/2011", "time string"="2:00:36 PM"}, {"Guppy X"=748.9963733952476, "Guppy Y"=688.3256488506693, "M3 X"=409.17066846139596, "M3 Y"=321.436565243555, "temp"=247.0, "date string"="9/19/2011", "time string"="2:01:37 PM"}, {"Guppy X"=752.2723856572197, "Guppy Y"=692.0461451454092, "M3 X"=409.6513442799375, "M3 Y"=321.1850598889393, "temp"=247.0, "date string"="9/19/2011", "time string"="2:02:37 PM"}, {"Guppy X"=752.2709912595651, "Guppy Y"=692.106541329599, "M3 X"=409.4546417138285, "M3 Y"=321.07292440589873, "temp"=247.0, "date string"="9/19/2011", "time string"="2:03:37 PM"}, {"Guppy X"=752.1109039702988, "Guppy Y"=692.0165595610434, "M3 X"=409.18224724528454, "M3 Y"=320.7215786061638, "temp"=247.0, "date string"="9/19/2011", "time string"="2:04:37 PM"}, {"Guppy X"=752.0995096674974, "Guppy Y"=692.0538106636852, "M3 X"=409.6673411234072, "M3 Y"=321.54673074178146, "temp"=247.0, "date string"="9/19/2011", "time string"="2:05:37 PM"}, {"Guppy X"=752.65670016994, "Guppy Y"=692.0066095766914, "M3 X"=409.0447680166018, "M3 Y"=321.6007283203871, "temp"=247.0, "date string"="9/19/2011", "time string"="2:06:37 PM"}, {"Guppy X"=752.9754210094104, "Guppy Y"=691.7227575329467, "M3 X"=405.0078079123815, "M3 Y"=321.562008646996, "temp"=248.0, "date string"="9/19/2011", "time string"="2:07:37 PM"}, {"Guppy X"=748.9290409968834, "Guppy Y"=688.7762489304198, "M3 X"=409.4853052115657, "M3 Y"=321.7700193877692, "temp"=247.0, "date string"="9/19/2011", "time string"="2:08:38 PM"}, {"Guppy X"=752.1197879257371, "Guppy Y"=692.3101759470595, "M3 X"=409.8106839058528, "M3 Y"=321.66686825253083, "temp"=247.0, "date string"="9/19/2011", "time string"="2:09:38 PM"}, {"Guppy X"=752.0903930580478, "Guppy Y"=692.2491445143218, "M3 X"=409.89302315770345, "M3 Y"=321.66210519731345, "temp"=247.0, "date string"="9/19/2011", "time string"="2:10:38 PM"}, {"Guppy X"=748.9504266300319, "Guppy Y"=688.7724780243406, "M3 X"=409.4272939195868, "M3 Y"=322.17842767166235, "temp"=247.0, "date string"="9/19/2011", "time string"="2:11:38 PM"}, {"Guppy X"=751.9658387822766, "Guppy Y"=692.198521195641, "M3 X"=410.10503077720574, "M3 Y"=321.55826868158744, "temp"=247.0, "date string"="9/19/2011", "time string"="2:12:38 PM"}, {"Guppy X"=752.6518252288198, "Guppy Y"=692.4981265966622, "M3 X"=410.25621164435904, "M3 Y"=322.9751675413792, "temp"=247.0, "date string"="9/19/2011", "time string"="2:13:38 PM"}, {"Guppy X"=752.2889650548483, "Guppy Y"=692.3658161327949, "M3 X"=408.5804600002017, "M3 Y"=321.8346270205321, "temp"=247.0, "date string"="9/19/2011", "time string"="2:14:38 PM"}, {"Guppy X"=752.4502394800579, "Guppy Y"=692.3266140326579, "M3 X"=409.3356446228491, "M3 Y"=321.70858881662485, "temp"=247.0, "date string"="9/19/2011", "time string"="2:15:38 PM"}, {"Guppy X"=752.51921505235, "Guppy Y"=692.4821230028404, "M3 X"=408.7587075374135, "M3 Y"=321.74774198020197, "temp"=247.0, "date string"="9/19/2011", "time string"="2:16:39 PM"}, {"Guppy X"=751.2404823688341, "Guppy Y"=691.2372140903133, "M3 X"=409.2700353312254, "M3 Y"=321.382643222989, "temp"=247.0, "date string"="9/19/2011", "time string"="2:17:39 PM"}, {"Guppy X"=752.1051606461699, "Guppy Y"=692.6020904577276, "M3 X"=410.2916783538149, "M3 Y"=321.72146705746576, "temp"=247.0, "date string"="9/19/2011", "time string"="2:18:39 PM"}, {"Guppy X"=752.1673577091269, "Guppy Y"=692.5212860048119, "M3 X"=410.26434856483564, "M3 Y"=321.3479363425704, "temp"=247.0, "date string"="9/19/2011", "time string"="2:19:39 PM"}, {"Guppy X"=752.2390523409604, "Guppy Y"=692.4710709243113, "M3 X"=410.32549790166235, "M3 Y"=321.0765201279923, "temp"=247.0, "date string"="9/19/2011", "time string"="2:20:39 PM"}, {"Guppy X"=751.9690698767449, "Guppy Y"=692.5170758753974, "M3 X"=410.07986676691985, "M3 Y"=321.010327141879, "temp"=247.0, "date string"="9/19/2011", "time string"="2:21:39 PM"}, {"Guppy X"=752.2042843124453, "Guppy Y"=692.4168716563507, "M3 X"=410.1743390480173, "M3 Y"=320.64734197243257, "temp"=247.0, "date string"="9/19/2011", "time string"="2:22:39 PM"}, {"Guppy X"=751.4617969779028, "Guppy Y"=692.5054781319429, "M3 X"=411.02573255725986, "M3 Y"=321.2196815626615, "temp"=247.0, "date string"="9/19/2011", "time string"="2:23:39 PM"}, {"Guppy X"=751.9120763839527, "Guppy Y"=692.564612779302, "M3 X"=410.26946266484816, "M3 Y"=321.24758317306487, "temp"=247.0, "date string"="9/19/2011", "time string"="2:24:39 PM"}, {"Guppy X"=752.1670895958721, "Guppy Y"=692.6165593091046, "M3 X"=407.850156871642, "M3 Y"=320.98883175892774, "temp"=247.0, "date string"="9/19/2011", "time string"="2:25:39 PM"}, {"Guppy X"=751.9516887623339, "Guppy Y"=692.9751771208219, "M3 X"=409.9509035076413, "M3 Y"=321.89691185059644, "temp"=247.0, "date string"="9/19/2011", "time string"="2:26:39 PM"}, {"Guppy X"=751.6856355199661, "Guppy Y"=692.6409328135173, "M3 X"=410.9923043082412, "M3 Y"=321.6585618805576, "temp"=247.0, "date string"="9/19/2011", "time string"="2:27:40 PM"}, {"Guppy X"=751.901299632035, "Guppy Y"=692.8009586118312, "M3 X"=410.6370879461895, "M3 Y"=321.7659765391012, "temp"=248.0, "date string"="9/19/2011", "time string"="2:28:40 PM"}, {"Guppy X"=751.81596469182, "Guppy Y"=692.660928943851, "M3 X"=410.86546389620617, "M3 Y"=321.10914395366655, "temp"=247.0, "date string"="9/19/2011", "time string"="2:29:40 PM"}, {"Guppy X"=751.6453292743429, "Guppy Y"=692.7966800372719, "M3 X"=411.1103816032697, "M3 Y"=320.927480018003, "temp"=247.0, "date string"="9/19/2011", "time string"="2:30:40 PM"}, {"Guppy X"=748.7584194898751, "Guppy Y"=689.307239529239, "M3 X"=410.3217960900149, "M3 Y"=321.4745571469458, "temp"=247.0, "date string"="9/19/2011", "time string"="2:31:40 PM"}, {"Guppy X"=751.8444940472881, "Guppy Y"=692.555041040163, "M3 X"=410.3779258264213, "M3 Y"=321.3318454499137, "temp"=247.0, "date string"="9/19/2011", "time string"="2:32:40 PM"}, {"Guppy X"=751.299881529499, "Guppy Y"=692.5405349470851, "M3 X"=411.39767154163906, "M3 Y"=321.2963374140681, "temp"=247.0, "date string"="9/19/2011", "time string"="2:33:40 PM"}, {"Guppy X"=751.7635773762057, "Guppy Y"=692.736664725469, "M3 X"=410.55524867596125, "M3 Y"=321.8083645353311, "temp"=247.0, "date string"="9/19/2011", "time string"="2:34:40 PM"}, {"Guppy X"=751.695491466281, "Guppy Y"=692.7905957056785, "M3 X"=410.4990603634014, "M3 Y"=321.9969677755017, "temp"=247.0, "date string"="9/19/2011", "time string"="2:35:40 PM"}, {"Guppy X"=751.6700691089565, "Guppy Y"=692.7845594446582, "M3 X"=410.78327867922934, "M3 Y"=321.41101176798486, "temp"=247.0, "date string"="9/19/2011", "time string"="2:36:40 PM"}, {"Guppy X"=751.9434874232869, "Guppy Y"=692.7271991613152, "M3 X"=410.49783685492014, "M3 Y"=321.3826639959425, "temp"=247.0, "date string"="9/19/2011", "time string"="2:37:41 PM"}, {"Guppy X"=751.6310414412883, "Guppy Y"=692.6512544314845, "M3 X"=412.13052977273617, "M3 Y"=322.52694543199993, "temp"=247.0, "date string"="9/19/2011", "time string"="2:38:41 PM"}, {"Guppy X"=751.6916350391831, "Guppy Y"=692.8073421001751, "M3 X"=410.91335130232574, "M3 Y"=321.0000042132186, "temp"=247.0, "date string"="9/19/2011", "time string"="2:39:41 PM"}, {"Guppy X"=751.881720393624, "Guppy Y"=692.9950513098483, "M3 X"=411.19637970584927, "M3 Y"=322.5430886150657, "temp"=247.0, "date string"="9/19/2011", "time string"="2:40:41 PM"}, {"Guppy X"=751.6388299391452, "Guppy Y"=693.1098714490842, "M3 X"=411.0860870861307, "M3 Y"=320.70978865123476, "temp"=247.0, "date string"="9/19/2011", "time string"="2:41:41 PM"}, {"Guppy X"=751.6237745819442, "Guppy Y"=693.1678856237476, "M3 X"=412.2360936569896, "M3 Y"=322.462684238137, "temp"=247.0, "date string"="9/19/2011", "time string"="2:42:41 PM"}, {"Guppy X"=751.7429238270594, "Guppy Y"=693.2560391596834, "M3 X"=410.8902003948849, "M3 Y"=321.05961973563103, "temp"=247.0, "date string"="9/19/2011", "time string"="2:43:41 PM"}, {"Guppy X"=751.8180604915932, "Guppy Y"=693.2429646026621, "M3 X"=410.9090495109282, "M3 Y"=321.1037361885751, "temp"=247.0, "date string"="9/19/2011", "time string"="2:44:41 PM"}, {"Guppy X"=751.5164351662723, "Guppy Y"=693.1728054029685, "M3 X"=411.56994998931583, "M3 Y"=321.06128637801646, "temp"=247.0, "date string"="9/19/2011", "time string"="2:45:41 PM"}, {"Guppy X"=746.9869814386495, "Guppy Y"=687.9568815381338, "M3 X"=411.08676449101506, "M3 Y"=321.0287465029143, "temp"=248.0, "date string"="9/19/2011", "time string"="2:46:41 PM"}, {"Guppy X"=750.5281918001624, "Guppy Y"=691.9927934488501, "M3 X"=411.30838309974, "M3 Y"=321.4231617556818, "temp"=247.0, "date string"="9/19/2011", "time string"="2:47:42 PM"}, {"Guppy X"=751.2622923832027, "Guppy Y"=693.1284683630887, "M3 X"=412.9062052586211, "M3 Y"=322.051798565576, "temp"=247.0, "date string"="9/19/2011", "time string"="2:48:42 PM"}, {"Guppy X"=751.7453688206928, "Guppy Y"=693.4051763383269, "M3 X"=411.4223008981489, "M3 Y"=321.15185433684275, "temp"=247.0, "date string"="9/19/2011", "time string"="2:49:42 PM"}, {"Guppy X"=751.2417511827529, "Guppy Y"=693.2117705734854, "M3 X"=412.1101398879473, "M3 Y"=320.6905775538397, "temp"=248.0, "date string"="9/19/2011", "time string"="2:50:42 PM"}, {"Guppy X"=nan, "Guppy Y"=nan, "M3 X"=nan, "M3 Y"=nan, "temp"=248.0, "date string"="9/19/2011", "time string"="2:51:42 PM"}, {"Guppy X"=751.5975875340971, "Guppy Y"=693.1283592887221, "M3 X"=411.15232970466894, "M3 Y"=320.699281776746, "temp"=247.0, "date string"="9/19/2011", "time string"="2:52:42 PM"}, {"Guppy X"=751.4296386258793, "Guppy Y"=693.443268422662, "M3 X"=411.2818405251548, "M3 Y"=320.77593553431853, "temp"=247.0, "date string"="9/19/2011", "time string"="2:53:42 PM"}, {"Guppy X"=751.7376293589815, "Guppy Y"=693.5351340918368, "M3 X"=411.23199642465283, "M3 Y"=320.6193001269333, "temp"=247.0, "date string"="9/19/2011", "time string"="2:54:42 PM"}, {"Guppy X"=751.2631755308927, "Guppy Y"=693.3120734791287, "M3 X"=412.2157593937993, "M3 Y"=320.45719865844956, "temp"=247.0, "date string"="9/19/2011", "time string"="2:55:42 PM"}, {"Guppy X"=751.7861650538636, "Guppy Y"=693.3895110104271, "M3 X"=412.71173125954584, "M3 Y"=322.14322010491384, "temp"=247.0, "date string"="9/19/2011", "time string"="2:56:42 PM"}, {"Guppy X"=751.5743402293639, "Guppy Y"=693.6622004162755, "M3 X"=411.61862769046144, "M3 Y"=321.49162475047183, "temp"=248.0, "date string"="9/19/2011", "time string"="2:57:42 PM"}, {"Guppy X"=751.2301338641015, "Guppy Y"=693.4758037801479, "M3 X"=412.26610059416635, "M3 Y"=321.13024223163376, "temp"=248.0, "date string"="9/19/2011", "time string"="2:58:42 PM"}, {"Guppy X"=751.3958121164345, "Guppy Y"=693.0597767168491, "M3 X"=410.7058532656337, "M3 Y"=320.5461593342578, "temp"=247.0, "date string"="9/19/2011", "time string"="2:59:43 PM"}, {"Guppy X"=751.0831283958272, "Guppy Y"=693.2825476679092, "M3 X"=413.6824388784167, "M3 Y"=321.9735461711453, "temp"=247.0, "date string"="9/19/2011", "time string"="3:00:43 PM"}, {"Guppy X"=751.5217020607993, "Guppy Y"=693.4446430986471, "M3 X"=411.8600102652084, "M3 Y"=320.6233262999365, "temp"=247.0, "date string"="9/19/2011", "time string"="3:01:43 PM"}, {"Guppy X"=751.2647542078025, "Guppy Y"=693.2656802275757, "M3 X"=412.2432509884069, "M3 Y"=320.02963687215936, "temp"=247.0, "date string"="9/19/2011", "time string"="3:02:43 PM"}, {"Guppy X"=751.1770769882395, "Guppy Y"=693.4499107684618, "M3 X"=412.3472118710066, "M3 Y"=320.3918919065887, "temp"=247.0, "date string"="9/19/2011", "time string"="3:03:43 PM"}, {"Guppy X"=751.2316903424066, "Guppy Y"=693.4348685119186, "M3 X"=412.0941463553365, "M3 Y"=320.60905487742747, "temp"=247.0, "date string"="9/19/2011", "time string"="3:04:43 PM"}, {"Guppy X"=751.7904004425309, "Guppy Y"=693.3535694112654, "M3 X"=411.3235353436704, "M3 Y"=320.24617898043414, "temp"=247.0, "date string"="9/19/2011", "time string"="3:05:43 PM"}, {"Guppy X"=751.0102733042605, "Guppy Y"=693.5614943675806, "M3 X"=412.5735630635852, "M3 Y"=320.49850390526245, "temp"=247.0, "date string"="9/19/2011", "time string"="3:06:43 PM"}, {"Guppy X"=751.1571043532166, "Guppy Y"=693.4197234760462, "M3 X"=412.2244651644907, "M3 Y"=320.63706033641694, "temp"=247.0, "date string"="9/19/2011", "time string"="3:07:43 PM"}, {"Guppy X"=751.397136049288, "Guppy Y"=693.5804266106893, "M3 X"=413.1983425097715, "M3 Y"=322.24628873226953, "temp"=247.0, "date string"="9/19/2011", "time string"="3:08:43 PM"}, {"Guppy X"=751.1813641907327, "Guppy Y"=693.5811938084255, "M3 X"=413.34346677698494, "M3 Y"=322.525854504386, "temp"=247.0, "date string"="9/19/2011", "time string"="3:09:43 PM"}, {"Guppy X"=751.1196923190934, "Guppy Y"=693.570602863972, "M3 X"=412.42234507875696, "M3 Y"=320.8207355924468, "temp"=247.0, "date string"="9/19/2011", "time string"="3:10:44 PM"}, {"Guppy X"=750.9816449837574, "Guppy Y"=693.7281411916053, "M3 X"=413.3312313872101, "M3 Y"=322.1474662557128, "temp"=247.0, "date string"="9/19/2011", "time string"="3:11:44 PM"}, {"Guppy X"=746.0769367015813, "Guppy Y"=688.4188518051968, "M3 X"=412.9231148444275, "M3 Y"=320.57997630152727, "temp"=247.0, "date string"="9/19/2011", "time string"="3:12:44 PM"}, {"Guppy X"=751.3398420976616, "Guppy Y"=693.8073969466933, "M3 X"=412.28054246880447, "M3 Y"=320.73542197499205, "temp"=247.0, "date string"="9/19/2011", "time string"="3:13:44 PM"}, {"Guppy X"=751.2802817278301, "Guppy Y"=693.6508460979785, "M3 X"=412.26771928364656, "M3 Y"=320.496149698954, "temp"=247.0, "date string"="9/19/2011", "time string"="3:14:44 PM"}, {"Guppy X"=751.015165268455, "Guppy Y"=693.5617163681137, "M3 X"=412.63109180258203, "M3 Y"=320.46205623195556, "temp"=247.0, "date string"="9/19/2011", "time string"="3:15:44 PM"}, {"Guppy X"=751.1172861957937, "Guppy Y"=693.5934735534527, "M3 X"=413.4878041398919, "M3 Y"=321.7641306662081, "temp"=247.0, "date string"="9/19/2011", "time string"="3:16:44 PM"}, {"Guppy X"=751.3812029817566, "Guppy Y"=693.8057988511487, "M3 X"=412.037870786816, "M3 Y"=320.55200692108315, "temp"=247.0, "date string"="9/19/2011", "time string"="3:17:44 PM"}, {"Guppy X"=751.0744792045264, "Guppy Y"=693.5966982242941, "M3 X"=412.8095374535378, "M3 Y"=320.0169355107555, "temp"=247.0, "date string"="9/19/2011", "time string"="3:18:45 PM"}, {"Guppy X"=749.6434422239314, "Guppy Y"=692.4445829189947, "M3 X"=412.3794812876626, "M3 Y"=320.3061526628607, "temp"=247.0, "date string"="9/19/2011", "time string"="3:19:45 PM"}, {"Guppy X"=751.0237527544358, "Guppy Y"=693.8231787149341, "M3 X"=412.08315040813875, "M3 Y"=320.3527290540405, "temp"=247.0, "date string"="9/19/2011", "time string"="3:20:45 PM"}, {"Guppy X"=750.9742298622141, "Guppy Y"=693.8192098646356, "M3 X"=412.1771661861317, "M3 Y"=320.3358506890576, "temp"=247.0, "date string"="9/19/2011", "time string"="3:21:45 PM"}, {"Guppy X"=750.9413104891603, "Guppy Y"=693.7126006541554, "M3 X"=412.898433742365, "M3 Y"=320.24260765797385, "temp"=247.0, "date string"="9/19/2011", "time string"="3:22:45 PM"}, {"Guppy X"=750.0592291753117, "Guppy Y"=692.5568307646287, "M3 X"=413.5169932119078, "M3 Y"=321.23066933727773, "temp"=247.0, "date string"="9/19/2011", "time string"="3:23:45 PM"}, {"Guppy X"=751.0920221524786, "Guppy Y"=693.8072062275625, "M3 X"=412.5271099554788, "M3 Y"=320.16420344618695, "temp"=247.0, "date string"="9/19/2011", "time string"="3:24:45 PM"}, {"Guppy X"=751.0393525413248, "Guppy Y"=693.6906275628118, "M3 X"=412.6168951818247, "M3 Y"=320.28089642233886, "temp"=247.0, "date string"="9/19/2011", "time string"="3:25:45 PM"}, {"Guppy X"=750.863898797219, "Guppy Y"=693.638593381945, "M3 X"=412.7228400462873, "M3 Y"=320.0241715687621, "temp"=247.0, "date string"="9/19/2011", "time string"="3:26:45 PM"}, {"Guppy X"=751.6136114588716, "Guppy Y"=693.5582146245041, "M3 X"=411.72781422643465, "M3 Y"=319.8479409858857, "temp"=247.0, "date string"="9/19/2011", "time string"="3:27:46 PM"}, {"Guppy X"=751.2667746380107, "Guppy Y"=693.6793295961039, "M3 X"=411.42521385673456, "M3 Y"=320.5709518893779, "temp"=247.0, "date string"="9/19/2011", "time string"="3:28:46 PM"}, {"Guppy X"=751.0968083852496, "Guppy Y"=693.7539656764446, "M3 X"=412.61459599665943, "M3 Y"=320.3398814564825, "temp"=247.0, "date string"="9/19/2011", "time string"="3:29:46 PM"}, {"Guppy X"=750.5247487319409, "Guppy Y"=693.7172020981714, "M3 X"=416.1113457545125, "M3 Y"=322.73812753440563, "temp"=246.0, "date string"="9/19/2011", "time string"="3:30:46 PM"}, {"Guppy X"=751.5085534568346, "Guppy Y"=693.9906626389508, "M3 X"=412.0858485617335, "M3 Y"=320.2871384186254, "temp"=247.0, "date string"="9/19/2011", "time string"="3:31:46 PM"}, {"Guppy X"=750.4925324665182, "Guppy Y"=693.7638522427958, "M3 X"=413.6634749876351, "M3 Y"=320.03666912131814, "temp"=247.0, "date string"="9/19/2011", "time string"="3:32:46 PM"}, {"Guppy X"=746.1984556019086, "Guppy Y"=688.8964874693271, "M3 X"=413.02591233375847, "M3 Y"=320.26282144701906, "temp"=247.0, "date string"="9/19/2011", "time string"="3:33:46 PM"}, {"Guppy X"=749.839887882212, "Guppy Y"=692.5493649360548, "M3 X"=412.79626656894743, "M3 Y"=320.11222172110087, "temp"=247.0, "date string"="9/19/2011", "time string"="3:34:46 PM"}, {"Guppy X"=750.865754364004, "Guppy Y"=693.9845666023728, "M3 X"=412.98745666863834, "M3 Y"=320.09478053347686, "temp"=247.0, "date string"="9/19/2011", "time string"="3:35:46 PM"}, {"Guppy X"=751.0813092342096, "Guppy Y"=693.986546118434, "M3 X"=412.60081629948587, "M3 Y"=320.10489295379926, "temp"=247.0, "date string"="9/19/2011", "time string"="3:36:46 PM"}, {"Guppy X"=751.269654182359, "Guppy Y"=693.8712567656078, "M3 X"=412.17447435518676, "M3 Y"=319.54793716355033, "temp"=247.0, "date string"="9/19/2011", "time string"="3:37:46 PM"}, {"Guppy X"=750.8885555792904, "Guppy Y"=694.0719467833013, "M3 X"=412.91390519996065, "M3 Y"=319.8386556376081, "temp"=247.0, "date string"="9/19/2011", "time string"="3:38:46 PM"}, {"Guppy X"=751.2056061989031, "Guppy Y"=693.8496304821085, "M3 X"=413.96203518707136, "M3 Y"=320.83831385805615, "temp"=247.0, "date string"="9/19/2011", "time string"="3:39:46 PM"}, {"Guppy X"=750.0432599411693, "Guppy Y"=692.8371408265712, "M3 X"=413.69953878269604, "M3 Y"=321.18750687452183, "temp"=247.0, "date string"="9/19/2011", "time string"="3:40:47 PM"}, {"Guppy X"=750.8173010169983, "Guppy Y"=694.0688463784161, "M3 X"=412.8701272409456, "M3 Y"=320.0984044287259, "temp"=247.0, "date string"="9/19/2011", "time string"="3:41:47 PM"}, {"Guppy X"=750.818275530509, "Guppy Y"=693.980214611825, "M3 X"=413.01058324838476, "M3 Y"=319.7617866139183, "temp"=247.0, "date string"="9/19/2011", "time string"="3:42:47 PM"}, {"Guppy X"=750.8411912612842, "Guppy Y"=693.812700241239, "M3 X"=412.9570355705766, "M3 Y"=319.3390041310186, "temp"=247.0, "date string"="9/19/2011", "time string"="3:43:47 PM"}, {"Guppy X"=750.9398040624965, "Guppy Y"=693.9102255533165, "M3 X"=412.86294828321337, "M3 Y"=319.3130412676993, "temp"=247.0, "date string"="9/19/2011", "time string"="3:44:47 PM"}, {"Guppy X"=751.1023856750554, "Guppy Y"=694.08346509262, "M3 X"=412.63321971935517, "M3 Y"=319.7111377850602, "temp"=247.0, "date string"="9/19/2011", "time string"="3:45:47 PM"}, {"Guppy X"=750.6354670486779, "Guppy Y"=694.0069568305483, "M3 X"=413.3169842244686, "M3 Y"=319.85293290096774, "temp"=247.0, "date string"="9/19/2011", "time string"="3:46:47 PM"}, {"Guppy X"=749.649293372754, "Guppy Y"=692.6890220438142, "M3 X"=413.22097118277094, "M3 Y"=319.6955740481307, "temp"=247.0, "date string"="9/19/2011", "time string"="3:47:47 PM"}, {"Guppy X"=750.7670458617033, "Guppy Y"=694.0154961876144, "M3 X"=413.090253240123, "M3 Y"=319.3211770411101, "temp"=247.0, "date string"="9/19/2011", "time string"="3:48:47 PM"}, {"Guppy X"=751.1682411158773, "Guppy Y"=694.0764119381529, "M3 X"=412.43959001451447, "M3 Y"=319.5095327932938, "temp"=247.0, "date string"="9/19/2011", "time string"="3:49:47 PM"}, {"Guppy X"=749.2239461802902, "Guppy Y"=691.5658179420811, "M3 X"=411.9558778587674, "M3 Y"=319.2942457720638, "temp"=247.0, "date string"="9/19/2011", "time string"="3:50:48 PM"}, {"Guppy X"=750.969931371546, "Guppy Y"=694.0816981533585, "M3 X"=414.98695287863086, "M3 Y"=321.95756947711476, "temp"=247.0, "date string"="9/19/2011", "time string"="3:51:48 PM"}, {"Guppy X"=751.348844057213, "Guppy Y"=694.070285780741, "M3 X"=412.1621415255337, "M3 Y"=319.4721248968697, "temp"=247.0, "date string"="9/19/2011", "time string"="3:52:48 PM"}, {"Guppy X"=750.998515955125, "Guppy Y"=694.0612454556428, "M3 X"=414.0179808810623, "M3 Y"=320.68112612699133, "temp"=247.0, "date string"="9/19/2011", "time string"="3:53:48 PM"}, {"Guppy X"=751.3986106365497, "Guppy Y"=694.3150359125871, "M3 X"=412.1113764461991, "M3 Y"=319.7053371747204, "temp"=247.0, "date string"="9/19/2011", "time string"="3:54:48 PM"}, {"Guppy X"=750.968932020632, "Guppy Y"=694.1023203351258, "M3 X"=413.8429042688437, "M3 Y"=320.5862416049313, "temp"=247.0, "date string"="9/19/2011", "time string"="3:55:48 PM"}, {"Guppy X"=750.6328172935276, "Guppy Y"=694.0274695313294, "M3 X"=413.5335965033023, "M3 Y"=318.8461789378958, "temp"=247.0, "date string"="9/19/2011", "time string"="3:56:48 PM"}, {"Guppy X"=750.8365889420924, "Guppy Y"=694.1193553586478, "M3 X"=412.570549378206, "M3 Y"=319.00469975823285, "temp"=247.0, "date string"="9/19/2011", "time string"="3:57:48 PM"}, {"Guppy X"=751.1029353900781, "Guppy Y"=694.523178672803, "M3 X"=412.4651445682111, "M3 Y"=319.515457900205, "temp"=247.0, "date string"="9/19/2011", "time string"="3:58:48 PM"}, {"Guppy X"=750.7974478350299, "Guppy Y"=694.1558603419872, "M3 X"=413.3995285042852, "M3 Y"=318.92854607600907, "temp"=247.0, "date string"="9/19/2011", "time string"="3:59:48 PM"}, {"Guppy X"=750.9928865946039, "Guppy Y"=694.2568572942212, "M3 X"=412.73266009837084, "M3 Y"=319.6274338603704, "temp"=247.0, "date string"="9/19/2011", "time string"="4:00:48 PM"}, {"Guppy X"=746.7834666163916, "Guppy Y"=689.136408612753, "M3 X"=412.318810326627, "M3 Y"=319.32941992080754, "temp"=247.0, "date string"="9/19/2011", "time string"="4:01:48 PM"}, {"Guppy X"=750.9924272711794, "Guppy Y"=694.0861147724937, "M3 X"=412.6719827882038, "M3 Y"=318.9965649821557, "temp"=247.0, "date string"="9/19/2011", "time string"="4:02:48 PM"}, {"Guppy X"=751.0421484593957, "Guppy Y"=694.380147369661, "M3 X"=412.3492701653418, "M3 Y"=319.5470899137111, "temp"=247.0, "date string"="9/19/2011", "time string"="4:03:49 PM"}, {"Guppy X"=748.7191709401512, "Guppy Y"=691.8172434777895, "M3 X"=413.53441662312184, "M3 Y"=320.69796512832494, "temp"=247.0, "date string"="9/19/2011", "time string"="4:04:49 PM"}, {"Guppy X"=751.2075133222119, "Guppy Y"=694.5939746318878, "M3 X"=412.01150270059884, "M3 Y"=319.7318928330481, "temp"=247.0, "date string"="9/19/2011", "time string"="4:05:49 PM"}, {"Guppy X"=750.5652880052858, "Guppy Y"=693.9304348606008, "M3 X"=413.83815174045856, "M3 Y"=319.3774888586741, "temp"=247.0, "date string"="9/19/2011", "time string"="4:06:49 PM"}, {"Guppy X"=750.9367127918935, "Guppy Y"=694.2925344367451, "M3 X"=412.6831540263581, "M3 Y"=319.7750226221045, "temp"=247.0, "date string"="9/19/2011", "time string"="4:07:49 PM"}, {"Guppy X"=751.1115522060352, "Guppy Y"=694.2963498461321, "M3 X"=413.3475913732734, "M3 Y"=321.3492622612698, "temp"=247.0, "date string"="9/19/2011", "time string"="4:08:49 PM"}, {"Guppy X"=749.8813776285087, "Guppy Y"=693.1359792702104, "M3 X"=412.356935502411, "M3 Y"=319.483134012611, "temp"=247.0, "date string"="9/19/2011", "time string"="4:09:49 PM"}, {"Guppy X"=751.0441651137019, "Guppy Y"=694.5916329257508, "M3 X"=412.3137446123849, "M3 Y"=320.068383477104, "temp"=247.0, "date string"="9/19/2011", "time string"="4:10:49 PM"}, {"Guppy X"=751.0791283045227, "Guppy Y"=694.6047902387163, "M3 X"=412.4787750108629, "M3 Y"=319.8244438918222, "temp"=247.0, "date string"="9/19/2011", "time string"="4:11:49 PM"}, {"Guppy X"=750.9592138733417, "Guppy Y"=694.637466954021, "M3 X"=412.99784296910997, "M3 Y"=319.4280253537373, "temp"=247.0, "date string"="9/19/2011", "time string"="4:12:49 PM"}, {"Guppy X"=750.8723626172996, "Guppy Y"=694.5444041224958, "M3 X"=412.9113544692276, "M3 Y"=318.95961826356415, "temp"=247.0, "date string"="9/19/2011", "time string"="4:13:49 PM"}, {"Guppy X"=750.267164036306, "Guppy Y"=694.2331174994115, "M3 X"=414.24357487558086, "M3 Y"=318.6140657934207, "temp"=247.0, "date string"="9/19/2011", "time string"="4:14:49 PM"}, {"Guppy X"=750.8105569815383, "Guppy Y"=694.5309750390378, "M3 X"=412.7689724097494, "M3 Y"=318.9594018985408, "temp"=247.0, "date string"="9/19/2011", "time string"="4:15:50 PM"}, {"Guppy X"=nan, "Guppy Y"=nan, "M3 X"=nan, "M3 Y"=nan, "temp"=247.0, "date string"="9/19/2011", "time string"="4:16:50 PM"}, {"Guppy X"=750.8319644474535, "Guppy Y"=694.6155354040928, "M3 X"=412.626898535494, "M3 Y"=319.2847338156111, "temp"=247.0, "date string"="9/19/2011", "time string"="4:17:50 PM"}, {"Guppy X"=751.0096116150256, "Guppy Y"=694.8189069182883, "M3 X"=412.3947200222655, "M3 Y"=319.16965142791327, "temp"=247.0, "date string"="9/19/2011", "time string"="4:18:50 PM"}, {"Guppy X"=749.5746062581618, "Guppy Y"=693.3235060506231, "M3 X"=412.85352616355857, "M3 Y"=319.17177945739536, "temp"=247.0, "date string"="9/19/2011", "time string"="4:19:50 PM"}, {"Guppy X"=750.4042500975401, "Guppy Y"=694.4464237614385, "M3 X"=413.16679677435417, "M3 Y"=319.0963513862932, "temp"=247.0, "date string"="9/19/2011", "time string"="4:20:50 PM"}, {"Guppy X"=749.7346413868204, "Guppy Y"=693.0727155226211, "M3 X"=413.1033437377524, "M3 Y"=318.41701339517624, "temp"=247.0, "date string"="9/19/2011", "time string"="4:21:50 PM"}, {"Guppy X"=750.6318118394779, "Guppy Y"=694.7049173052084, "M3 X"=413.10320432416995, "M3 Y"=318.5249591771171, "temp"=247.0, "date string"="9/19/2011", "time string"="4:22:50 PM"}, {"Guppy X"=750.9167946708844, "Guppy Y"=694.884465406247, "M3 X"=413.8877186137434, "M3 Y"=320.07978951401384, "temp"=247.0, "date string"="9/19/2011", "time string"="4:23:51 PM"}, {"Guppy X"=750.75812789489, "Guppy Y"=694.6247141842334, "M3 X"=413.1944764519587, "M3 Y"=318.4676428287867, "temp"=247.0, "date string"="9/19/2011", "time string"="4:24:51 PM"}, {"Guppy X"=750.6415856543568, "Guppy Y"=694.6896719600393, "M3 X"=413.13616075476244, "M3 Y"=318.59917344531067, "temp"=247.0, "date string"="9/19/2011", "time string"="4:25:51 PM"}, {"Guppy X"=751.2738787006841, "Guppy Y"=694.650016905453, "M3 X"=412.12175166438317, "M3 Y"=318.4720084518622, "temp"=247.0, "date string"="9/19/2011", "time string"="4:26:51 PM"}, {"Guppy X"=751.5398786198825, "Guppy Y"=694.662732314265, "M3 X"=411.76608075316545, "M3 Y"=318.71038735961815, "temp"=247.0, "date string"="9/19/2011", "time string"="4:27:51 PM"}, {"Guppy X"=750.9651612547651, "Guppy Y"=694.679261827501, "M3 X"=412.5333677884105, "M3 Y"=318.7473897494635, "temp"=247.0, "date string"="9/19/2011", "time string"="4:28:51 PM"}, {"Guppy X"=750.9960634407659, "Guppy Y"=694.8255001521275, "M3 X"=411.81251317477745, "M3 Y"=318.5861197119753, "temp"=247.0, "date string"="9/19/2011", "time string"="4:29:51 PM"}, {"Guppy X"=750.2566302192112, "Guppy Y"=693.4964680985931, "M3 X"=412.12844139533587, "M3 Y"=318.4530205078832, "temp"=247.0, "date string"="9/19/2011", "time string"="4:30:51 PM"}, {"Guppy X"=751.2278318385044, "Guppy Y"=694.9342885350206, "M3 X"=412.0643607796003, "M3 Y"=318.0078433771081, "temp"=247.0, "date string"="9/19/2011", "time string"="4:31:51 PM"}, {"Guppy X"=751.017804958786, "Guppy Y"=694.9214223983817, "M3 X"=412.8193133387178, "M3 Y"=318.04194834988573, "temp"=247.0, "date string"="9/19/2011", "time string"="4:32:51 PM"}, {"Guppy X"=750.9467914421598, "Guppy Y"=695.0394723755484, "M3 X"=411.8870575171001, "M3 Y"=318.8900107948704, "temp"=247.0, "date string"="9/19/2011", "time string"="4:33:51 PM"}, {"Guppy X"=751.2157903491478, "Guppy Y"=694.7833199858312, "M3 X"=412.2018587329942, "M3 Y"=318.31990963790554, "temp"=247.0, "date string"="9/19/2011", "time string"="4:34:52 PM"}, {"Guppy X"=751.4291429052228, "Guppy Y"=694.9830662196158, "M3 X"=411.76831342993387, "M3 Y"=318.7921295314075, "temp"=247.0, "date string"="9/19/2011", "time string"="4:35:52 PM"}, {"Guppy X"=750.9836727325908, "Guppy Y"=694.9538360222334, "M3 X"=412.5346483738608, "M3 Y"=318.59055441289524, "temp"=247.0, "date string"="9/19/2011", "time string"="4:36:52 PM"}, {"Guppy X"=751.1024896903153, "Guppy Y"=694.6249214731365, "M3 X"=412.5981318444654, "M3 Y"=318.1469614771005, "temp"=247.0, "date string"="9/19/2011", "time string"="4:37:52 PM"}, {"Guppy X"=751.4977846031182, "Guppy Y"=694.8300789456576, "M3 X"=411.7073576616193, "M3 Y"=318.192624944076, "temp"=247.0, "date string"="9/19/2011", "time string"="4:38:52 PM"}, {"Guppy X"=751.5256415788618, "Guppy Y"=694.9249979824609, "M3 X"=411.2610328454229, "M3 Y"=318.3247686433629, "temp"=247.0, "date string"="9/19/2011", "time string"="4:39:52 PM"}, {"Guppy X"=751.1352006292894, "Guppy Y"=694.6293553246812, "M3 X"=413.6621194538754, "M3 Y"=319.36046154647437, "temp"=247.0, "date string"="9/19/2011", "time string"="4:40:52 PM"}, {"Guppy X"=751.4457185339434, "Guppy Y"=694.6617109435055, "M3 X"=411.53368270044183, "M3 Y"=318.1237720582787, "temp"=247.0, "date string"="9/19/2011", "time string"="4:41:52 PM"}, {"Guppy X"=750.7143545486779, "Guppy Y"=694.6104883928567, "M3 X"=412.220301920337, "M3 Y"=318.38531541314273, "temp"=247.0, "date string"="9/19/2011", "time string"="4:42:52 PM"}, {"Guppy X"=750.9655545079455, "Guppy Y"=694.8342320037466, "M3 X"=412.58994732111825, "M3 Y"=318.30813784834976, "temp"=247.0, "date string"="9/19/2011", "time string"="4:43:53 PM"}, {"Guppy X"=751.541526802546, "Guppy Y"=695.0118100550142, "M3 X"=411.4177262385268, "M3 Y"=318.41596308181767, "temp"=247.0, "date string"="9/19/2011", "time string"="4:44:53 PM"}, {"Guppy X"=751.2086173757884, "Guppy Y"=695.0607284784884, "M3 X"=411.6807619568996, "M3 Y"=318.1021749653595, "temp"=247.0, "date string"="9/19/2011", "time string"="4:45:53 PM"}, {"Guppy X"=751.1417383759695, "Guppy Y"=694.8323363835963, "M3 X"=412.62764651902256, "M3 Y"=317.97823549157994, "temp"=247.0, "date string"="9/19/2011", "time string"="4:46:53 PM"}, {"Guppy X"=751.2655465609045, "Guppy Y"=695.2147220354504, "M3 X"=411.9385757854042, "M3 Y"=318.11814111042304, "temp"=247.0, "date string"="9/19/2011", "time string"="4:47:53 PM"}, {"Guppy X"=751.190362179009, "Guppy Y"=695.0992081673427, "M3 X"=412.23544960257993, "M3 Y"=317.5839213110551, "temp"=247.0, "date string"="9/19/2011", "time string"="4:48:53 PM"}, {"Guppy X"=751.0118484108566, "Guppy Y"=695.0714179656129, "M3 X"=412.3599008552943, "M3 Y"=318.01130814649844, "temp"=247.0, "date string"="9/19/2011", "time string"="4:49:53 PM"}, {"Guppy X"=751.0450377755338, "Guppy Y"=694.924452788502, "M3 X"=413.0067795288867, "M3 Y"=317.51450675899207, "temp"=247.0, "date string"="9/19/2011", "time string"="4:50:53 PM"}, {"Guppy X"=746.7639856079653, "Guppy Y"=689.6660167152288, "M3 X"=411.4352092913014, "M3 Y"=317.708622815031, "temp"=247.0, "date string"="9/19/2011", "time string"="4:51:53 PM"}, {"Guppy X"=749.9826626850012, "Guppy Y"=693.674784033613, "M3 X"=412.2640563809424, "M3 Y"=317.8814556674849, "temp"=247.0, "date string"="9/19/2011", "time string"="4:52:54 PM"}, {"Guppy X"=751.3690363389908, "Guppy Y"=694.6802565488982, "M3 X"=412.41346635746453, "M3 Y"=317.1227538613287, "temp"=247.0, "date string"="9/19/2011", "time string"="4:53:54 PM"}, {"Guppy X"=751.6190883467013, "Guppy Y"=695.2970273731025, "M3 X"=411.14455973316024, "M3 Y"=317.4092390410734, "temp"=247.0, "date string"="9/19/2011", "time string"="4:54:54 PM"}, {"Guppy X"=750.8079464602455, "Guppy Y"=695.0907050077307, "M3 X"=411.97454069721294, "M3 Y"=316.7928729903538, "temp"=246.0, "date string"="9/19/2011", "time string"="4:55:54 PM"}, {"Guppy X"=750.8618788213171, "Guppy Y"=695.0556731796913, "M3 X"=412.4750075257008, "M3 Y"=317.2340339551414, "temp"=247.0, "date string"="9/19/2011", "time string"="4:56:54 PM"}, {"Guppy X"=749.0180921746608, "Guppy Y"=692.4033963635987, "M3 X"=411.61584898434563, "M3 Y"=317.2215998291644, "temp"=247.0, "date string"="9/19/2011", "time string"="4:57:54 PM"}, {"Guppy X"=751.164875679493, "Guppy Y"=695.112785818504, "M3 X"=414.64202445107014, "M3 Y"=320.1517299827713, "temp"=247.0, "date string"="9/19/2011", "time string"="4:58:54 PM"}, {"Guppy X"=751.2058230959688, "Guppy Y"=695.3858985304669, "M3 X"=411.9562650113716, "M3 Y"=317.8208909993843, "temp"=247.0, "date string"="9/19/2011", "time string"="4:59:55 PM"}, {"Guppy X"=750.8026245792186, "Guppy Y"=694.8454107045916, "M3 X"=412.984154222402, "M3 Y"=317.76551478177595, "temp"=246.0, "date string"="9/19/2011", "time string"="5:00:55 PM"}, {"Guppy X"=751.295618490877, "Guppy Y"=695.2741032286897, "M3 X"=411.6928478773503, "M3 Y"=317.69744042286897, "temp"=247.0, "date string"="9/19/2011", "time string"="5:01:55 PM"}, {"Guppy X"=751.1409591645596, "Guppy Y"=695.4727707426489, "M3 X"=412.1325087184559, "M3 Y"=317.76493767780954, "temp"=240.0, "date string"="9/19/2011", "time string"="5:02:55 PM"}, {"Guppy X"=746.1362995813556, "Guppy Y"=690.052714772838, "M3 X"=412.40493855957965, "M3 Y"=317.86108375529426, "temp"=247.0, "date string"="9/19/2011", "time string"="5:03:55 PM"}, {"Guppy X"=751.1676965929488, "Guppy Y"=695.2894329807738, "M3 X"=412.39606080532883, "M3 Y"=317.69159463411677, "temp"=247.0, "date string"="9/19/2011", "time string"="5:04:55 PM"}, {"Guppy X"=750.4264636941855, "Guppy Y"=695.10326806191, "M3 X"=413.31411798356817, "M3 Y"=317.28597382949533, "temp"=247.0, "date string"="9/19/2011", "time string"="5:05:55 PM"}, {"Guppy X"=750.7899056284856, "Guppy Y"=695.4210863061841, "M3 X"=412.5484885106708, "M3 Y"=317.78612051716766, "temp"=247.0, "date string"="9/19/2011", "time string"="5:06:55 PM"}, {"Guppy X"=751.0448841157589, "Guppy Y"=695.3658032674571, "M3 X"=411.87975384536304, "M3 Y"=317.9289701107647, "temp"=247.0, "date string"="9/19/2011", "time string"="5:07:55 PM"}, {"Guppy X"=750.9223746527433, "Guppy Y"=695.2683171809991, "M3 X"=412.50923447399543, "M3 Y"=317.28178275255, "temp"=247.0, "date string"="9/19/2011", "time string"="5:08:55 PM"}, {"Guppy X"=750.9594002826392, "Guppy Y"=695.3222640431732, "M3 X"=412.22805324799515, "M3 Y"=317.6921868245069, "temp"=247.0, "date string"="9/19/2011", "time string"="5:09:56 PM"}, {"Guppy X"=750.8770307057171, "Guppy Y"=695.3495751479053, "M3 X"=413.6166900084817, "M3 Y"=318.70156911911874, "temp"=247.0, "date string"="9/19/2011", "time string"="5:10:56 PM"}, {"Guppy X"=751.2667822995182, "Guppy Y"=695.4486300858403, "M3 X"=411.80786580509135, "M3 Y"=317.5524418704044, "temp"=247.0, "date string"="9/19/2011", "time string"="5:11:56 PM"}, {"Guppy X"=749.9384718566182, "Guppy Y"=693.9848850994623, "M3 X"=412.3091390150142, "M3 Y"=317.17286969345537, "temp"=247.0, "date string"="9/19/2011", "time string"="5:12:56 PM"}, {"Guppy X"=751.0421218248902, "Guppy Y"=695.483122918636, "M3 X"=412.4170921311021, "M3 Y"=316.992581186587, "temp"=247.0, "date string"="9/19/2011", "time string"="5:13:56 PM"}, {"Guppy X"=751.2062271946126, "Guppy Y"=695.1560450841359, "M3 X"=411.92640490839426, "M3 Y"=316.7688486056487, "temp"=247.0, "date string"="9/19/2011", "time string"="5:14:56 PM"}, {"Guppy X"=751.803495071321, "Guppy Y"=695.1106542216361, "M3 X"=411.09365602316234, "M3 Y"=316.89345331693636, "temp"=247.0, "date string"="9/19/2011", "time string"="5:15:56 PM"}, {"Guppy X"=750.7961151669715, "Guppy Y"=695.2780031262503, "M3 X"=412.48268967812567, "M3 Y"=317.4029492832117, "temp"=247.0, "date string"="9/19/2011", "time string"="5:16:56 PM"}, {"Guppy X"=750.2549778068442, "Guppy Y"=694.1220358279078, "M3 X"=411.94186911191815, "M3 Y"=317.4565674899177, "temp"=247.0, "date string"="9/19/2011", "time string"="5:17:56 PM"}, {"Guppy X"=751.1664944877159, "Guppy Y"=695.6354947168834, "M3 X"=411.9256125074825, "M3 Y"=317.7584501432272, "temp"=246.0, "date string"="9/19/2011", "time string"="5:18:57 PM"}, {"Guppy X"=750.8764695637967, "Guppy Y"=695.5346932927553, "M3 X"=412.54385373525463, "M3 Y"=317.6957007963548, "temp"=247.0, "date string"="9/19/2011", "time string"="5:19:57 PM"}, {"Guppy X"=748.353330119227, "Guppy Y"=693.0578218782655, "M3 X"=411.8672504438762, "M3 Y"=317.150540260367, "temp"=247.0, "date string"="9/19/2011", "time string"="5:20:57 PM"}, {"Guppy X"=750.7505804028377, "Guppy Y"=695.5221541249269, "M3 X"=412.49551646364927, "M3 Y"=317.1802051287759, "temp"=247.0, "date string"="9/19/2011", "time string"="5:21:57 PM"}, {"Guppy X"=750.849896073297, "Guppy Y"=695.5125429656433, "M3 X"=413.3614182143303, "M3 Y"=318.76568306262953, "temp"=247.0, "date string"="9/19/2011", "time string"="5:22:57 PM"}, {"Guppy X"=751.2694265897935, "Guppy Y"=695.5964292197765, "M3 X"=411.8111949508682, "M3 Y"=317.3065313945435, "temp"=247.0, "date string"="9/19/2011", "time string"="5:23:57 PM"}, {"Guppy X"=751.0028550135247, "Guppy Y"=695.6843480191142, "M3 X"=412.51479993285557, "M3 Y"=317.7034908437815, "temp"=247.0, "date string"="9/19/2011", "time string"="5:24:57 PM"}, {"Guppy X"=750.4439053180072, "Guppy Y"=695.333276618156, "M3 X"=412.8569624525819, "M3 Y"=317.2715448160002, "temp"=247.0, "date string"="9/19/2011", "time string"="5:25:57 PM"}, {"Guppy X"=751.1009985634777, "Guppy Y"=695.7311058376044, "M3 X"=411.52694854261654, "M3 Y"=317.91253484088725, "temp"=247.0, "date string"="9/19/2011", "time string"="5:26:57 PM"}, {"Guppy X"=750.9699120290412, "Guppy Y"=695.5809611683953, "M3 X"=412.4047992876061, "M3 Y"=317.92605866142344, "temp"=247.0, "date string"="9/19/2011", "time string"="5:27:57 PM"}, {"Guppy X"=744.3658981238821, "Guppy Y"=688.1539132928851, "M3 X"=412.4908586275594, "M3 Y"=317.91836297287267, "temp"=247.0, "date string"="9/19/2011", "time string"="5:28:58 PM"}, {"Guppy X"=750.1234675919056, "Guppy Y"=694.6219690575458, "M3 X"=412.22245653013033, "M3 Y"=317.7348633521124, "temp"=247.0, "date string"="9/19/2011", "time string"="5:29:58 PM"}, {"Guppy X"=751.0813153015935, "Guppy Y"=695.6704439385054, "M3 X"=412.26789303035804, "M3 Y"=317.34256273569076, "temp"=246.0, "date string"="9/19/2011", "time string"="5:30:58 PM"}, {"Guppy X"=751.5091224713093, "Guppy Y"=695.9102640961588, "M3 X"=411.47370683628776, "M3 Y"=317.5708811145518, "temp"=247.0, "date string"="9/19/2011", "time string"="5:31:58 PM"}, {"Guppy X"=750.9420145168906, "Guppy Y"=695.4560688418068, "M3 X"=413.20566535626284, "M3 Y"=317.16168510057514, "temp"=247.0, "date string"="9/19/2011", "time string"="5:32:58 PM"}, {"Guppy X"=750.76728573001, "Guppy Y"=695.4330308950081, "M3 X"=413.03858080076066, "M3 Y"=316.94565189950106, "temp"=247.0, "date string"="9/19/2011", "time string"="5:33:58 PM"}, {"Guppy X"=750.8941105992794, "Guppy Y"=695.9467238476315, "M3 X"=412.4573406482924, "M3 Y"=317.13625201751705, "temp"=246.0, "date string"="9/19/2011", "time string"="5:34:58 PM"}, {"Guppy X"=751.1794950461979, "Guppy Y"=695.8246320528924, "M3 X"=413.21341125707147, "M3 Y"=318.5418716689865, "temp"=246.0, "date string"="9/19/2011", "time string"="5:35:58 PM"}, {"Guppy X"=750.9620166459043, "Guppy Y"=695.8134363099849, "M3 X"=412.30849104361, "M3 Y"=317.00953574373847, "temp"=247.0, "date string"="9/19/2011", "time string"="5:36:58 PM"}, {"Guppy X"=751.0714414501605, "Guppy Y"=695.5605402530588, "M3 X"=412.186694767561, "M3 Y"=317.3447619618632, "temp"=247.0, "date string"="9/19/2011", "time string"="5:37:59 PM"}, {"Guppy X"=750.8461632979993, "Guppy Y"=695.5241527968369, "M3 X"=nan, "M3 Y"=nan, "temp"=247.0, "date string"="9/19/2011", "time string"="5:38:59 PM"}, {"Guppy X"=750.8317575081528, "Guppy Y"=695.8253206789736, "M3 X"=412.776164202755, "M3 Y"=317.1903984244865, "temp"=247.0, "date string"="9/19/2011", "time string"="5:39:59 PM"}, {"Guppy X"=750.5859357394148, "Guppy Y"=695.6388651992918, "M3 X"=413.23024629403034, "M3 Y"=317.1079275489414, "temp"=247.0, "date string"="9/19/2011", "time string"="5:40:59 PM"}]
  in  "datalog path (use dialog)":path=path "C:/Temp/TEMPPOS.DAT"
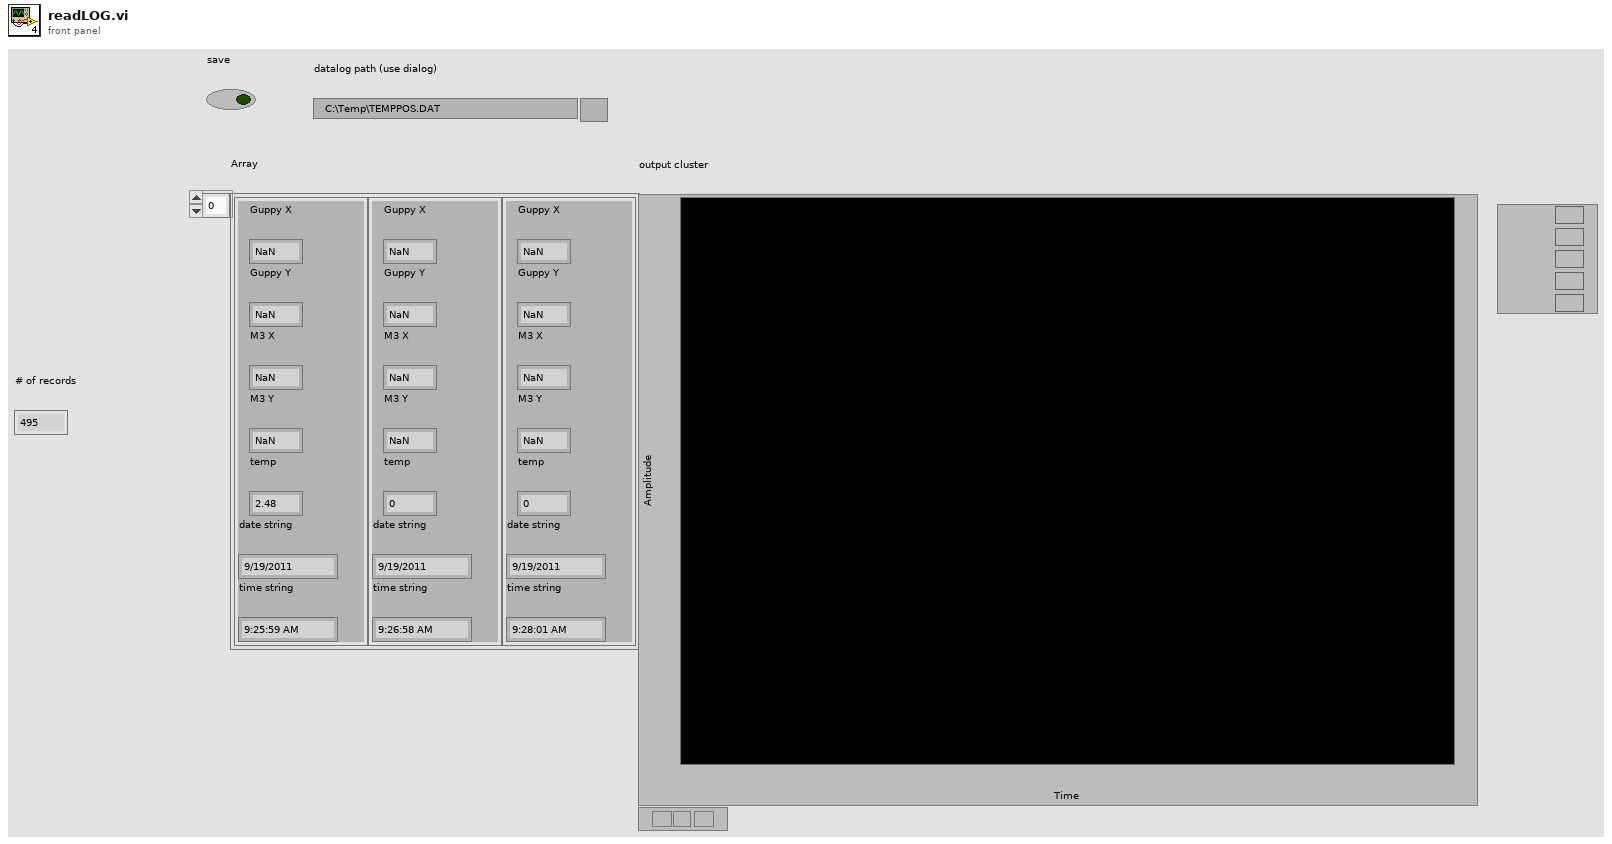
[diagram p1: front panel]
types:
  T1 = cluster{"Guppy X":dbl, "Guppy Y":dbl, "M3 X":dbl, "M3 Y":dbl, "temp":dbl, "date string":string, "time string":string}[]
  T2 = cluster{"Guppy X":dbl, "Guppy Y":dbl, "M3 X":dbl, "M3 Y":dbl, "temp":dbl, "date string":string, "time string":string}
  T3 = enum16{"open", "replace", "create", "open or create", "replace or create", "replace or create with confirmation"}
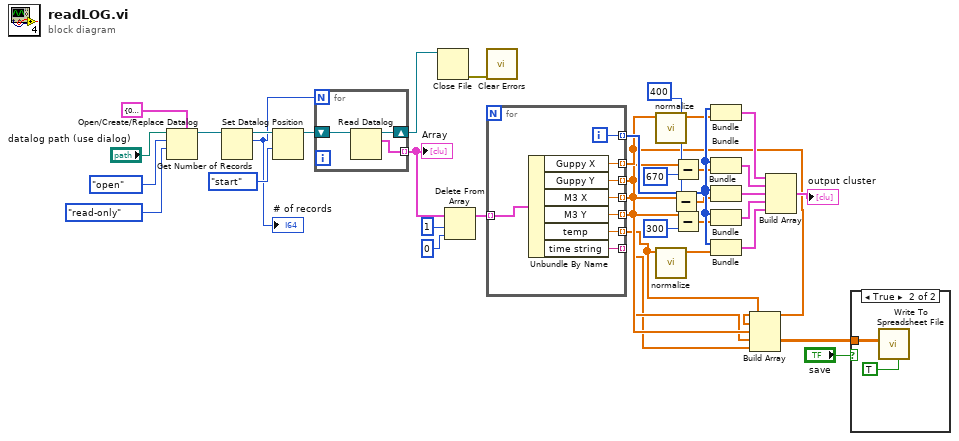
[diagram p0: block diagram]
diagram:
  n1 = Open/Create/Replace Datalog(5:T2 {"Guppy X"=0.0, "Guppy Y"=0.0, "M3 X"=0.0, "M3 Y"=0.0, "temp"=0.0, "date string"="", "time string"=""} ("cluster"), 9:enum16{"read/write", "read-only", "write-only"}."read-only" ("access (0:read/write)"), 10:T3."open" ("operation (0:open)"), 11:"datalog path (use dialog)") -> (3:w28:refnum<k1>)  [unwired: 2 in, 2 out]
  n2 = Get Number of Records(7:w28) -> (2:w30:i64, 3:w32:refnum<k1>)  [unwired: 1 in, 1 out]
  "# of records" <- w30
  n3 = Set Datalog Position(5:enum16{"start", "end", "current"}."start" ("from (0:start)"), 7:w32) -> (3:w31:refnum<k1>)  [unwired: 2 in, 1 out]
  n4 = for {
    N: w30 -> [_]
    shift-right: [w39] -> w29
    shift-left: w31 -> [w40]
    tunnel: [w38] -> w26 mode=indexing
    n5 = Read Datalog(7:w40) -> (2:w38:T2, 3:w39:refnum<k1>)  [unwired: 2 in, 1 out]
  }
  "Array" <- w26
  n6 = Close File(refnum=w29) -> (error out=w34:errorcluster)  [unwired: 1 in, 1 out]
  n7 = Delete From Array(array=w26, length=1, index=0) -> (array with subset deleted=w23:T1)  [unwired: 1 out]
  n8 = call <vilib>:"Clear Errors.vi"("error in (no error)"=w34) -> ()  [unwired: 6 in, 1 out]
  n9 = for {
    tunnel: w23 -> [w48] mode=indexing
    tunnel: [w47] -> w7 mode=indexing
    tunnel: [w46] -> w6 mode=indexing
    tunnel: [w45] -> w5 mode=indexing
    tunnel: [w44] -> w4 mode=indexing
    tunnel: [w43] -> w2 mode=indexing
    tunnel: [w42] -> w22 mode=indexing
    tunnel: [w41] -> _ mode=indexing
    i -> [w42]
    n10 = Unbundle By Name(w48) -> ("Guppy X"=w47:dbl, "Guppy Y"=w46:dbl, "M3 X"=w45:dbl, "M3 Y"=w44:dbl, "temp"=w43:dbl, "time string"=w41:string)
  }
  n11 = call "normalize.vi"("Array in"=w7) -> ("Array out"=w16:dbl[])  [unwired: 10 in]
  n12 = call "normalize.vi"("Array in"=w2) -> ("Array out"=w15:dbl[])  [unwired: 10 in]
  n13 = Subtract(x=w5, y=400 ("M3 X")) -> (x-y=w9:dbl[])
  n14 = Subtract(x=w6, y=670) -> (x-y=w13:dbl[])
  n15 = Subtract(x=w4, y=300) -> (x-y=w12:dbl[])
  n16 = Bundle(w22, "Array out"=w16) -> (w21:cluster{i32[], "Array out":dbl[]})  [unwired: 1 in]
  n17 = Bundle(w22, w13) -> (w20:cluster{i32[], dbl[]})  [unwired: 1 in]
  n18 = Bundle(w22, w9) -> (w8:cluster{i32[], dbl[]})  [unwired: 1 in]
  n19 = Bundle(w22, w12) -> (w19:cluster{i32[], dbl[]})  [unwired: 1 in]
  n20 = Bundle(w22, "Array out"=w15) -> (w18:cluster{i32[], "Array out":dbl[]})  [unwired: 1 in]
  n21 = Build Array(w2, w7, w6, w5, w4) -> (w3:dbl[][])
  n22 = Build Array(w21, w20, w8, w19, w18) -> (→"output cluster":cluster{i32[], "Array out":dbl[]}[])
  n23 = case shown="True" "save" {
    tunnel: w3 -> [_ w50]
    frame False {
    }
    frame True {
      n24 = call-poly <vilib>:"Write To Spreadsheet File.vi"("transpose? (no:F)"=TRUE, "2D data"=w50) -> ()  [unwired: 6 in, 1 out]
    }
  }
